vi "Tausand AB1000 Acquisition Example.vi"() -> ()   [LabVIEW 2015]
doc: "Example of a complete acquisition system using a Tausand Abacus.\n\nIncludes device identification, live settings changes and live data reading.\nData is shown in tables, graphs and saved in plain text files.\nUses a producer-consumer design pattern."
uses:
  <instrlib>/Tausand AB1000/Examples/sub vi/connectionState.ctl
  <instrlib>/Tausand AB1000/Public/Controls/settings4ch.ctl
  <instrlib>/Tausand AB1000/Public/Controls/configMultipleCoincRing.ctl
  <instrlib>/Tausand AB1000/Examples/sub vi/defaultSettings.ctl
  <instrlib>/Tausand AB1000/Public/Controls/deviceTypeRing.ctl
  <instrlib>/Tausand AB1000/Public/Controls/settings2ch.ctl
  <instrlib>/Tausand AB1000/Public/Controls/counters2ch.ctl
  <instrlib>/Tausand AB1000/Public/Controls/counters4ch.ctl
  <vilib>/Utility/miscctls.llb/LVRowAndColumnUnsignedTypeDef.ctl
  <instrlib>/Tausand AB1000/Public/Controls/channelRing.ctl
  <vilib>/Utility/file.llb/Write Delimited Spreadsheet (string).vi
  <vilib>/Utility/file.llb/Read Delimited Spreadsheet (string).vi
  <instrlib>/Tausand AB1000/Tausand AB1000.lvlib
panel:
  out "ref ctrls":T1
  out "timer-settings 2":timestamp
  in  "butLoadDefSett":bool
  out "ref indics":T2
  out "dafafile header":string[](array[string])
  in  "settings 2ch":T3={"sampling"=1000, "coincidence_window"=10, "delay_A"=0, "delay_B"=0, "sleep_A"=0, "sleep_B"=0} {"sleep_B" max=100 step=5; "sleep_A" max=100 step=5; "delay_B" max=100 step=5; "delay_A" max=100 step=5; "coincidence_window" min=1 max=50000 step=5; "sampling" items=["1ms"=1, "2ms"=2, "5ms"=5, "10ms"=10, "20ms"=20, "50ms"=50, "100ms"=100, "200ms"=200, "500ms"=500, "1s"=1000, "2s"=2000, "5s"=5000, "10s"=10000, "20s"=20000, "50s"=50000, "100s"=100000, "200s"=200000, "500s"=500000, "1000s"=1000000]}
  in  "settings 4ch":T4={"sampling"=1000, "coincidence_window"=10, "delay_A"=0, "delay_B"=0, "delay_C"=0, "delay_D"=0, "sleep_A"=0, "sleep_B"=0, "sleep_C"=0, "sleep_D"=0, "config_multiple_1"=240} {"config_multiple_1" items=["ABC"=224, "ABD"=208, "ACD"=176, "BCD"=112, "ABCD"=240]; "sleep_D" max=100 step=5; "sleep_C" max=100 step=5; "sleep_B" max=100 step=5; "sleep_A" max=100 step=5; "delay_D" max=100 step=5; "delay_C" max=100 step=5; "delay_B" max=100 step=5; "delay_A" max=100 step=5; "coincidence_window" min=1 max=10000 step=5; "sampling" items=["1ms"=1, "2ms"=2, "3ms"=3, "4ms"=4, "5ms"=5, "6ms"=6, "7ms"=7, "8ms"=8, "9ms"=9, "10ms"=10, "11ms"=11, "12ms"=12, "13ms"=13, "14ms"=14, "15ms"=15, "16ms"=16, "17ms"=17, "18ms"=18, "19ms"=19, "20ms"=20, "21ms"=21, "22ms"=22, "23ms"=23, "24ms"=24, "25ms"=25, "26ms"=26, "27ms"=27, "28ms"=28, "29ms"=29, "30ms"=30, "31ms"=31, "32ms"=32, "33ms"=33, "34ms"=34, "35ms"=35, "36ms"=36, "37ms"=37, "38ms"=38, "39ms"=39, "40ms"=40, "41ms"=41, "42ms"=42, "43ms"=43, "44ms"=44, "45ms"=45, "46ms"=46, "47ms"=47, "48ms"=48, "49ms"=49, "50ms"=50, "51ms"=51, "52ms"=52, "53ms"=53, "54ms"=54, "55ms"=55, "56ms"=56, "57ms"=57, "58ms"=58, "59ms"=59, "60ms"=60, "61ms"=61, "62ms"=62, "63ms"=63, "64ms"=64, "65ms"=65, "66ms"=66, "67ms"=67, "68ms"=68, "69ms"=69, "70ms"=70, "71ms"=71, "72ms"=72, "73ms"=73, "74ms"=74, "75ms"=75, "76ms"=76, "77ms"=77, "78ms"=78, "79ms"=79, "80ms"=80, "81ms"=81, "82ms"=82, "83ms"=83, "84ms"=84, "85ms"=85, "86ms"=86, "87ms"=87, "88ms"=88, "89ms"=89, "90ms"=90, "91ms"=91, "92ms"=92, "93ms"=93, "94ms"=94, "95ms"=95, "96ms"=96, "97ms"=97, "98ms"=98, "99ms"=99, "100ms"=100, "110ms"=110, "120ms"=120, "130ms"=130, "140ms"=140, "150ms"=150, "160ms"=160, "170ms"=170, "180ms"=180, "190ms"=190, "200ms"=200, "210ms"=210, "220ms"=220, "230ms"=230, "240ms"=240, "250ms"=250, "260ms"=260, "270ms"=270, "280ms"=280, "290ms"=290, "300ms"=300, "310ms"=310, "320ms"=320, "330ms"=330, "340ms"=340, "350ms"=350, "360ms"=360, "370ms"=370, "380ms"=380, "390ms"=390, "400ms"=400, "410ms"=410, "420ms"=420, "430ms"=430, "440ms"=440, "450ms"=450, "460ms"=460, "470ms"=470, "480ms"=480, "490ms"=490, "500ms"=500, "510ms"=510, "520ms"=520, "530ms"=530, "540ms"=540, "550ms"=550, "560ms"=560, "570ms"=570, "580ms"=580, "590ms"=590, "600ms"=600, "610ms"=610, "620ms"=620, "630ms"=630, "640ms"=640, "650ms"=650, "660ms"=660, "670ms"=670, "680ms"=680, "690ms"=690, "700ms"=700, "710ms"=710, "720ms"=720, "730ms"=730, "740ms"=740, "750ms"=750, "760ms"=760, "770ms"=770, "780ms"=780, "790ms"=790, "800ms"=800, "810ms"=810, "820ms"=820, "830ms"=830, "840ms"=840, "850ms"=850, "860ms"=860, "870ms"=870, "880ms"=880, "890ms"=890, "900ms"=900, "910ms"=910, "920ms"=920, "930ms"=930, "940ms"=940, "950ms"=950, "960ms"=960, "970ms"=970, "980ms"=980, "990ms"=990, "1,0s"=1000, "1,1s"=1100, "1,2s"=1200, "1,3s"=1300, "1,4s"=1400, "1,5s"=1500, "1,6s"=1600, "1,7s"=1700, "1,8s"=1800, "1,9s"=1900, "2,0s"=2000, "2,1s"=2100, "2,2s"=2200, "2,3s"=2300, "2,4s"=2400, "2,5s"=2500, "2,6s"=2600, "2,7s"=2700, "2,8s"=2800, "2,9s"=2900, "3,0s"=3000, "3,1s"=3100, "3,2s"=3200, "3,3s"=3300, "3,4s"=3400, "3,5s"=3500, "3,6s"=3600, "3,7s"=3700, "3,8s"=3800, "3,9s"=3900, "4,0s"=4000, "4,1s"=4100, "4,2s"=4200, "4,3s"=4300, "4,4s"=4400, "4,5s"=4500, "4,6s"=4600, "4,7s"=4700, "4,8s"=4800, "4,9s"=4900, "5,0s"=5000, "5,1s"=5100, "5,2s"=5200, "5,3s"=5300, "5,4s"=5400, "5,5s"=5500, "5,6s"=5600, "5,7s"=5700, "5,8s"=5800, "5,9s"=5900, "6,0s"=6000, "6,1s"=6100, "6,2s"=6200, "6,3s"=6300, "6,4s"=6400, "6,5s"=6500, "6,6s"=6600, "6,7s"=6700, "6,8s"=6800, "6,9s"=6900, "7,0s"=7000, "7,1s"=7100, "7,2s"=7200, "7,3s"=7300, "7,4s"=7400, "7,5s"=7500, "7,6s"=7600, "7,7s"=7700, "7,8s"=7800, "7,9s"=7900, "8,0s"=8000, "8,1s"=8100, "8,2s"=8200, "8,3s"=8300, "8,4s"=8400, "8,5s"=8500, "8,6s"=8600, "8,7s"=8700, "8,8s"=8800, "8,9s"=8900, "9,0s"=9000, "9,1s"=9100, "9,2s"=9200, "9,3s"=9300, "9,4s"=9400, "9,5s"=9500, "9,6s"=9600, "9,7s"=9700, "9,8s"=9800, "9,9s"=9900, "10s"=10000, "11s"=11000, "12s"=12000, "13s"=13000, "14s"=14000, "15s"=15000, "16s"=16000, "17s"=17000, "18s"=18000, "19s"=19000, "20s"=20000, "21s"=21000, "22s"=22000, "23s"=23000, "24s"=24000, "25s"=25000, "26s"=26000, "27s"=27000, "28s"=28000, "29s"=29000, "30s"=30000, "31s"=31000, "32s"=32000, "33s"=33000, "34s"=34000, "35s"=35000, "36s"=36000, "37s"=37000, "38s"=38000, "39s"=39000, "40s"=40000, "41s"=41000, "42s"=42000, "43s"=43000, "44s"=44000, "45s"=45000, "46s"=46000, "47s"=47000, "48s"=48000, "49s"=49000, "50s"=50000, "51s"=51000, "52s"=52000, "53s"=53000, "54s"=54000, "55s"=55000, "56s"=56000, "57s"=57000, "58s"=58000, "59s"=59000, "60s"=60000, "61s"=61000, "62s"=62000, "63s"=63000, "64s"=64000, "65s"=65000, "66s"=66000, "67s"=67000, "68s"=68000, "69s"=69000, "70s"=70000, "71s"=71000, "72s"=72000, "73s"=73000, "74s"=74000, "75s"=75000, "76s"=76000, "77s"=77000, "78s"=78000, "79s"=79000, "80s"=80000, "81s"=81000, "82s"=82000, "83s"=83000, "84s"=84000, "85s"=85000, "86s"=86000, "87s"=87000, "88s"=88000, "89s"=89000, "90s"=90000, "91s"=91000, "92s"=92000, "93s"=93000, "94s"=94000, "95s"=95000, "96s"=96000, "97s"=97000, "98s"=98000, "99s"=99000, "100s"=100000, "110s"=110000, "120s"=120000, "130s"=130000, "140s"=140000, "150s"=150000, "160s"=160000, "170s"=170000, "180s"=180000, "190s"=190000, "200s"=200000, "210s"=210000, "220s"=220000, "230s"=230000, "240s"=240000, "250s"=250000, "260s"=260000, "270s"=270000, "280s"=280000, "290s"=290000, "300s"=300000, "310s"=310000, "320s"=320000, "330s"=330000, "340s"=340000, "350s"=350000, "360s"=360000, "370s"=370000, "380s"=380000, "390s"=390000, "400s"=400000, "410s"=410000, "420s"=420000, "430s"=430000, "440s"=440000, "450s"=450000, "460s"=460000, "470s"=470000, "480s"=480000, "490s"=490000, "500s"=500000, "510s"=510000, "520s"=520000, "530s"=530000, "540s"=540000, "550s"=550000, "560s"=560000, "570s"=570000, "580s"=580000, "590s"=590000, "600s"=600000, "610s"=610000, "620s"=620000, "630s"=630000, "640s"=640000, "650s"=650000, "660s"=660000, "670s"=670000, "680s"=680000, "690s"=690000, "700s"=700000, "710s"=710000, "720s"=720000, "730s"=730000, "740s"=740000, "750s"=750000, "760s"=760000, "770s"=770000, "780s"=780000, "790s"=790000, "800s"=800000, "810s"=810000, "820s"=820000, "830s"=830000, "840s"=840000, "850s"=850000, "860s"=860000, "870s"=870000, "880s"=880000, "890s"=890000, "900s"=900000, "910s"=910000, "920s"=920000, "930s"=930000, "940s"=940000, "950s"=950000, "960s"=960000, "970s"=970000, "980s"=980000, "990s"=990000, "1000s"=1000000]}
  out "device type":T6 items=["any"=0, "AB1002"=1002, "AB1004"=1004, "AB1502"=1502, "AB1504"=1504, "AB2002"=2002, "AB2004"=2004, "AB2502"=2502, "AB2504"=2504]
  out "path-defsettings":path
  out "delimiter":string
  out "default settings":T7={"autogenerate"=FALSE, "datetime"=FALSE, "from_device"=FALSE, "directory"="", "file_prefix"="", "settings_suffix"="", "delimiter"="", "extension"="", "Abacus settings"={"sampling"=0, "coincidence_window"=0, "delay_A"=0, "delay_B"=0, "delay_C"=0, "delay_D"=0, "sleep_A"=0, "sleep_B"=0, "sleep_C"=0, "sleep_D"=0, "config_multiple_1"=240}} {"Abacus settings"."config_multiple_1" items=["ABC"=224, "ABD"=208, "ACD"=176, "BCD"=112, "ABCD"=240]; "Abacus settings"."sleep_D" max=100 step=5; "Abacus settings"."sleep_C" max=100 step=5; "Abacus settings"."sleep_B" max=100 step=5; "Abacus settings"."sleep_A" max=100 step=5; "Abacus settings"."delay_D" max=100 step=5; "Abacus settings"."delay_C" max=100 step=5; "Abacus settings"."delay_B" max=100 step=5; "Abacus settings"."delay_A" max=100 step=5; "Abacus settings"."coincidence_window" min=5 max=10000 step=5; "Abacus settings"."sampling" items=["1ms"=1, "2ms"=2, "3ms"=3, "4ms"=4, "5ms"=5, "6ms"=6, "7ms"=7, "8ms"=8, "9ms"=9, "10ms"=10, "11ms"=11, "12ms"=12, "13ms"=13, "14ms"=14, "15ms"=15, "16ms"=16, "17ms"=17, "18ms"=18, "19ms"=19, "20ms"=20, "21ms"=21, "22ms"=22, "23ms"=23, "24ms"=24, "25ms"=25, "26ms"=26, "27ms"=27, "28ms"=28, "29ms"=29, "30ms"=30, "31ms"=31, "32ms"=32, "33ms"=33, "34ms"=34, "35ms"=35, "36ms"=36, "37ms"=37, "38ms"=38, "39ms"=39, "40ms"=40, "41ms"=41, "42ms"=42, "43ms"=43, "44ms"=44, "45ms"=45, "46ms"=46, "47ms"=47, "48ms"=48, "49ms"=49, "50ms"=50, "51ms"=51, "52ms"=52, "53ms"=53, "54ms"=54, "55ms"=55, "56ms"=56, "57ms"=57, "58ms"=58, "59ms"=59, "60ms"=60, "61ms"=61, "62ms"=62, "63ms"=63, "64ms"=64, "65ms"=65, "66ms"=66, "67ms"=67, "68ms"=68, "69ms"=69, "70ms"=70, "71ms"=71, "72ms"=72, "73ms"=73, "74ms"=74, "75ms"=75, "76ms"=76, "77ms"=77, "78ms"=78, "79ms"=79, "80ms"=80, "81ms"=81, "82ms"=82, "83ms"=83, "84ms"=84, "85ms"=85, "86ms"=86, "87ms"=87, "88ms"=88, "89ms"=89, "90ms"=90, "91ms"=91, "92ms"=92, "93ms"=93, "94ms"=94, "95ms"=95, "96ms"=96, "97ms"=97, "98ms"=98, "99ms"=99, "100ms"=100, "110ms"=110, "120ms"=120, "130ms"=130, "140ms"=140, "150ms"=150, "160ms"=160, "170ms"=170, "180ms"=180, "190ms"=190, "200ms"=200, "210ms"=210, "220ms"=220, "230ms"=230, "240ms"=240, "250ms"=250, "260ms"=260, "270ms"=270, "280ms"=280, "290ms"=290, "300ms"=300, "310ms"=310, "320ms"=320, "330ms"=330, "340ms"=340, "350ms"=350, "360ms"=360, "370ms"=370, "380ms"=380, "390ms"=390, "400ms"=400, "410ms"=410, "420ms"=420, "430ms"=430, "440ms"=440, "450ms"=450, "460ms"=460, "470ms"=470, "480ms"=480, "490ms"=490, "500ms"=500, "510ms"=510, "520ms"=520, "530ms"=530, "540ms"=540, "550ms"=550, "560ms"=560, "570ms"=570, "580ms"=580, "590ms"=590, "600ms"=600, "610ms"=610, "620ms"=620, "630ms"=630, "640ms"=640, "650ms"=650, "660ms"=660, "670ms"=670, "680ms"=680, "690ms"=690, "700ms"=700, "710ms"=710, "720ms"=720, "730ms"=730, "740ms"=740, "750ms"=750, "760ms"=760, "770ms"=770, "780ms"=780, "790ms"=790, "800ms"=800, "810ms"=810, "820ms"=820, "830ms"=830, "840ms"=840, "850ms"=850, "860ms"=860, "870ms"=870, "880ms"=880, "890ms"=890, "900ms"=900, "910ms"=910, "920ms"=920, "930ms"=930, "940ms"=940, "950ms"=950, "960ms"=960, "970ms"=970, "980ms"=980, "990ms"=990, "1,0s"=1000, "1,1s"=1100, "1,2s"=1200, "1,3s"=1300, "1,4s"=1400, "1,5s"=1500, "1,6s"=1600, "1,7s"=1700, "1,8s"=1800, "1,9s"=1900, "2,0s"=2000, "2,1s"=2100, "2,2s"=2200, "2,3s"=2300, "2,4s"=2400, "2,5s"=2500, "2,6s"=2600, "2,7s"=2700, "2,8s"=2800, "2,9s"=2900, "3,0s"=3000, "3,1s"=3100, "3,2s"=3200, "3,3s"=3300, "3,4s"=3400, "3,5s"=3500, "3,6s"=3600, "3,7s"=3700, "3,8s"=3800, "3,9s"=3900, "4,0s"=4000, "4,1s"=4100, "4,2s"=4200, "4,3s"=4300, "4,4s"=4400, "4,5s"=4500, "4,6s"=4600, "4,7s"=4700, "4,8s"=4800, "4,9s"=4900, "5,0s"=5000, "5,1s"=5100, "5,2s"=5200, "5,3s"=5300, "5,4s"=5400, "5,5s"=5500, "5,6s"=5600, "5,7s"=5700, "5,8s"=5800, "5,9s"=5900, "6,0s"=6000, "6,1s"=6100, "6,2s"=6200, "6,3s"=6300, "6,4s"=6400, "6,5s"=6500, "6,6s"=6600, "6,7s"=6700, "6,8s"=6800, "6,9s"=6900, "7,0s"=7000, "7,1s"=7100, "7,2s"=7200, "7,3s"=7300, "7,4s"=7400, "7,5s"=7500, "7,6s"=7600, "7,7s"=7700, "7,8s"=7800, "7,9s"=7900, "8,0s"=8000, "8,1s"=8100, "8,2s"=8200, "8,3s"=8300, "8,4s"=8400, "8,5s"=8500, "8,6s"=8600, "8,7s"=8700, "8,8s"=8800, "8,9s"=8900, "9,0s"=9000, "9,1s"=9100, "9,2s"=9200, "9,3s"=9300, "9,4s"=9400, "9,5s"=9500, "9,6s"=9600, "9,7s"=9700, "9,8s"=9800, "9,9s"=9900, "10s"=10000, "11s"=11000, "12s"=12000, "13s"=13000, "14s"=14000, "15s"=15000, "16s"=16000, "17s"=17000, "18s"=18000, "19s"=19000, "20s"=20000, "21s"=21000, "22s"=22000, "23s"=23000, "24s"=24000, "25s"=25000, "26s"=26000, "27s"=27000, "28s"=28000, "29s"=29000, "30s"=30000, "31s"=31000, "32s"=32000, "33s"=33000, "34s"=34000, "35s"=35000, "36s"=36000, "37s"=37000, "38s"=38000, "39s"=39000, "40s"=40000, "41s"=41000, "42s"=42000, "43s"=43000, "44s"=44000, "45s"=45000, "46s"=46000, "47s"=47000, "48s"=48000, "49s"=49000, "50s"=50000, "51s"=51000, "52s"=52000, "53s"=53000, "54s"=54000, "55s"=55000, "56s"=56000, "57s"=57000, "58s"=58000, "59s"=59000, "60s"=60000, "61s"=61000, "62s"=62000, "63s"=63000, "64s"=64000, "65s"=65000, "66s"=66000, "67s"=67000, "68s"=68000, "69s"=69000, "70s"=70000, "71s"=71000, "72s"=72000, "73s"=73000, "74s"=74000, "75s"=75000, "76s"=76000, "77s"=77000, "78s"=78000, "79s"=79000, "80s"=80000, "81s"=81000, "82s"=82000, "83s"=83000, "84s"=84000, "85s"=85000, "86s"=86000, "87s"=87000, "88s"=88000, "89s"=89000, "90s"=90000, "91s"=91000, "92s"=92000, "93s"=93000, "94s"=94000, "95s"=95000, "96s"=96000, "97s"=97000, "98s"=98000, "99s"=99000, "100s"=100000, "110s"=110000, "120s"=120000, "130s"=130000, "140s"=140000, "150s"=150000, "160s"=160000, "170s"=170000, "180s"=180000, "190s"=190000, "200s"=200000, "210s"=210000, "220s"=220000, "230s"=230000, "240s"=240000, "250s"=250000, "260s"=260000, "270s"=270000, "280s"=280000, "290s"=290000, "300s"=300000, "310s"=310000, "320s"=320000, "330s"=330000, "340s"=340000, "350s"=350000, "360s"=360000, "370s"=370000, "380s"=380000, "390s"=390000, "400s"=400000, "410s"=410000, "420s"=420000, "430s"=430000, "440s"=440000, "450s"=450000, "460s"=460000, "470s"=470000, "480s"=480000, "490s"=490000, "500s"=500000, "510s"=510000, "520s"=520000, "530s"=530000, "540s"=540000, "550s"=550000, "560s"=560000, "570s"=570000, "580s"=580000, "590s"=590000, "600s"=600000, "610s"=610000, "620s"=620000, "630s"=630000, "640s"=640000, "650s"=650000, "660s"=660000, "670s"=670000, "680s"=680000, "690s"=690000, "700s"=700000, "710s"=710000, "720s"=720000, "730s"=730000, "740s"=740000, "750s"=750000, "760s"=760000, "770s"=770000, "780s"=780000, "790s"=790000, "800s"=800000, "810s"=810000, "820s"=820000, "830s"=830000, "840s"=840000, "850s"=850000, "860s"=860000, "870s"=870000, "880s"=880000, "890s"=890000, "900s"=900000, "910s"=910000, "920s"=920000, "930s"=930000, "940s"=940000, "950s"=950000, "960s"=960000, "970s"=970000, "980s"=980000, "990s"=990000, "1000s"=1000000]}
  out "settings_old":T4={"sampling"=1000, "coincidence_window"=10, "delay_A"=0, "delay_B"=0, "delay_C"=0, "delay_D"=0, "sleep_A"=0, "sleep_B"=0, "sleep_C"=0, "sleep_D"=0, "config_multiple_1"=0} {"config_multiple_1" items=["ABC"=224, "ABD"=208, "ACD"=176, "BCD"=112, "ABCD"=240]; "sleep_D" max=100 step=1; "sleep_C" max=100 step=1; "sleep_B" max=100 step=1; "sleep_A" max=100 step=1; "delay_D" max=100 step=1; "delay_C" max=100 step=1; "delay_B" max=100 step=1; "delay_A" max=100 step=1; "coincidence_window" min=1 max=10000 step=1; "sampling" items=["1ms"=1, "2ms"=2, "3ms"=3, "4ms"=4, "5ms"=5, "6ms"=6, "7ms"=7, "8ms"=8, "9ms"=9, "10ms"=10, "11ms"=11, "12ms"=12, "13ms"=13, "14ms"=14, "15ms"=15, "16ms"=16, "17ms"=17, "18ms"=18, "19ms"=19, "20ms"=20, "21ms"=21, "22ms"=22, "23ms"=23, "24ms"=24, "25ms"=25, "26ms"=26, "27ms"=27, "28ms"=28, "29ms"=29, "30ms"=30, "31ms"=31, "32ms"=32, "33ms"=33, "34ms"=34, "35ms"=35, "36ms"=36, "37ms"=37, "38ms"=38, "39ms"=39, "40ms"=40, "41ms"=41, "42ms"=42, "43ms"=43, "44ms"=44, "45ms"=45, "46ms"=46, "47ms"=47, "48ms"=48, "49ms"=49, "50ms"=50, "51ms"=51, "52ms"=52, "53ms"=53, "54ms"=54, "55ms"=55, "56ms"=56, "57ms"=57, "58ms"=58, "59ms"=59, "60ms"=60, "61ms"=61, "62ms"=62, "63ms"=63, "64ms"=64, "65ms"=65, "66ms"=66, "67ms"=67, "68ms"=68, "69ms"=69, "70ms"=70, "71ms"=71, "72ms"=72, "73ms"=73, "74ms"=74, "75ms"=75, "76ms"=76, "77ms"=77, "78ms"=78, "79ms"=79, "80ms"=80, "81ms"=81, "82ms"=82, "83ms"=83, "84ms"=84, "85ms"=85, "86ms"=86, "87ms"=87, "88ms"=88, "89ms"=89, "90ms"=90, "91ms"=91, "92ms"=92, "93ms"=93, "94ms"=94, "95ms"=95, "96ms"=96, "97ms"=97, "98ms"=98, "99ms"=99, "100ms"=100, "110ms"=110, "120ms"=120, "130ms"=130, "140ms"=140, "150ms"=150, "160ms"=160, "170ms"=170, "180ms"=180, "190ms"=190, "200ms"=200, "210ms"=210, "220ms"=220, "230ms"=230, "240ms"=240, "250ms"=250, "260ms"=260, "270ms"=270, "280ms"=280, "290ms"=290, "300ms"=300, "310ms"=310, "320ms"=320, "330ms"=330, "340ms"=340, "350ms"=350, "360ms"=360, "370ms"=370, "380ms"=380, "390ms"=390, "400ms"=400, "410ms"=410, "420ms"=420, "430ms"=430, "440ms"=440, "450ms"=450, "460ms"=460, "470ms"=470, "480ms"=480, "490ms"=490, "500ms"=500, "510ms"=510, "520ms"=520, "530ms"=530, "540ms"=540, "550ms"=550, "560ms"=560, "570ms"=570, "580ms"=580, "590ms"=590, "600ms"=600, "610ms"=610, "620ms"=620, "630ms"=630, "640ms"=640, "650ms"=650, "660ms"=660, "670ms"=670, "680ms"=680, "690ms"=690, "700ms"=700, "710ms"=710, "720ms"=720, "730ms"=730, "740ms"=740, "750ms"=750, "760ms"=760, "770ms"=770, "780ms"=780, "790ms"=790, "800ms"=800, "810ms"=810, "820ms"=820, "830ms"=830, "840ms"=840, "850ms"=850, "860ms"=860, "870ms"=870, "880ms"=880, "890ms"=890, "900ms"=900, "910ms"=910, "920ms"=920, "930ms"=930, "940ms"=940, "950ms"=950, "960ms"=960, "970ms"=970, "980ms"=980, "990ms"=990, "1,0s"=1000, "1,1s"=1100, "1,2s"=1200, "1,3s"=1300, "1,4s"=1400, "1,5s"=1500, "1,6s"=1600, "1,7s"=1700, "1,8s"=1800, "1,9s"=1900, "2,0s"=2000, "2,1s"=2100, "2,2s"=2200, "2,3s"=2300, "2,4s"=2400, "2,5s"=2500, "2,6s"=2600, "2,7s"=2700, "2,8s"=2800, "2,9s"=2900, "3,0s"=3000, "3,1s"=3100, "3,2s"=3200, "3,3s"=3300, "3,4s"=3400, "3,5s"=3500, "3,6s"=3600, "3,7s"=3700, "3,8s"=3800, "3,9s"=3900, "4,0s"=4000, "4,1s"=4100, "4,2s"=4200, "4,3s"=4300, "4,4s"=4400, "4,5s"=4500, "4,6s"=4600, "4,7s"=4700, "4,8s"=4800, "4,9s"=4900, "5,0s"=5000, "5,1s"=5100, "5,2s"=5200, "5,3s"=5300, "5,4s"=5400, "5,5s"=5500, "5,6s"=5600, "5,7s"=5700, "5,8s"=5800, "5,9s"=5900, "6,0s"=6000, "6,1s"=6100, "6,2s"=6200, "6,3s"=6300, "6,4s"=6400, "6,5s"=6500, "6,6s"=6600, "6,7s"=6700, "6,8s"=6800, "6,9s"=6900, "7,0s"=7000, "7,1s"=7100, "7,2s"=7200, "7,3s"=7300, "7,4s"=7400, "7,5s"=7500, "7,6s"=7600, "7,7s"=7700, "7,8s"=7800, "7,9s"=7900, "8,0s"=8000, "8,1s"=8100, "8,2s"=8200, "8,3s"=8300, "8,4s"=8400, "8,5s"=8500, "8,6s"=8600, "8,7s"=8700, "8,8s"=8800, "8,9s"=8900, "9,0s"=9000, "9,1s"=9100, "9,2s"=9200, "9,3s"=9300, "9,4s"=9400, "9,5s"=9500, "9,6s"=9600, "9,7s"=9700, "9,8s"=9800, "9,9s"=9900, "10s"=10000, "11s"=11000, "12s"=12000, "13s"=13000, "14s"=14000, "15s"=15000, "16s"=16000, "17s"=17000, "18s"=18000, "19s"=19000, "20s"=20000, "21s"=21000, "22s"=22000, "23s"=23000, "24s"=24000, "25s"=25000, "26s"=26000, "27s"=27000, "28s"=28000, "29s"=29000, "30s"=30000, "31s"=31000, "32s"=32000, "33s"=33000, "34s"=34000, "35s"=35000, "36s"=36000, "37s"=37000, "38s"=38000, "39s"=39000, "40s"=40000, "41s"=41000, "42s"=42000, "43s"=43000, "44s"=44000, "45s"=45000, "46s"=46000, "47s"=47000, "48s"=48000, "49s"=49000, "50s"=50000, "51s"=51000, "52s"=52000, "53s"=53000, "54s"=54000, "55s"=55000, "56s"=56000, "57s"=57000, "58s"=58000, "59s"=59000, "60s"=60000, "61s"=61000, "62s"=62000, "63s"=63000, "64s"=64000, "65s"=65000, "66s"=66000, "67s"=67000, "68s"=68000, "69s"=69000, "70s"=70000, "71s"=71000, "72s"=72000, "73s"=73000, "74s"=74000, "75s"=75000, "76s"=76000, "77s"=77000, "78s"=78000, "79s"=79000, "80s"=80000, "81s"=81000, "82s"=82000, "83s"=83000, "84s"=84000, "85s"=85000, "86s"=86000, "87s"=87000, "88s"=88000, "89s"=89000, "90s"=90000, "91s"=91000, "92s"=92000, "93s"=93000, "94s"=94000, "95s"=95000, "96s"=96000, "97s"=97000, "98s"=98000, "99s"=99000, "100s"=100000, "110s"=110000, "120s"=120000, "130s"=130000, "140s"=140000, "150s"=150000, "160s"=160000, "170s"=170000, "180s"=180000, "190s"=190000, "200s"=200000, "210s"=210000, "220s"=220000, "230s"=230000, "240s"=240000, "250s"=250000, "260s"=260000, "270s"=270000, "280s"=280000, "290s"=290000, "300s"=300000, "310s"=310000, "320s"=320000, "330s"=330000, "340s"=340000, "350s"=350000, "360s"=360000, "370s"=370000, "380s"=380000, "390s"=390000, "400s"=400000, "410s"=410000, "420s"=420000, "430s"=430000, "440s"=440000, "450s"=450000, "460s"=460000, "470s"=470000, "480s"=480000, "490s"=490000, "500s"=500000, "510s"=510000, "520s"=520000, "530s"=530000, "540s"=540000, "550s"=550000, "560s"=560000, "570s"=570000, "580s"=580000, "590s"=590000, "600s"=600000, "610s"=610000, "620s"=620000, "630s"=630000, "640s"=640000, "650s"=650000, "660s"=660000, "670s"=670000, "680s"=680000, "690s"=690000, "700s"=700000, "710s"=710000, "720s"=720000, "730s"=730000, "740s"=740000, "750s"=750000, "760s"=760000, "770s"=770000, "780s"=780000, "790s"=790000, "800s"=800000, "810s"=810000, "820s"=820000, "830s"=830000, "840s"=840000, "850s"=850000, "860s"=860000, "870s"=870000, "880s"=880000, "890s"=890000, "900s"=900000, "910s"=910000, "920s"=920000, "930s"=930000, "940s"=940000, "950s"=950000, "960s"=960000, "970s"=970000, "980s"=980000, "990s"=990000, "1000s"=1000000]}
  out "sttgs changed?":bool[](array[boolean])
  out "connection state":T8
  out "timer-reconnect":timestamp
  out "status":string
  out "path-new":path
  out "error":errorcluster
  out "path-settingsOld":path
  out "path-settings":path
  out "timer-settings":timestamp
  out "timer-readRequest":timestamp
  in  "Tab Control":T9(tab)
  out "dataTable":string[][](table)
  out "counters 2ch":T10
  out "counters 4ch":T11
  out "graph-A":cluster{timestamp[], u32[]}(graph) caption="small graph A"
  out "graph-B":cluster{timestamp[], u32[]}(graph) caption="small graph B"
  out "graph-C":cluster{timestamp[], u32[]}(graph) caption="small graph C"
  out "graph-D":cluster{timestamp[], u32[]}(graph) caption="small graph D"
  out "graph coinc":cluster{timestamp[], u32[]}[](graph)
  out "graph-A-S":cluster{timestamp[], u32[]}(graph) caption="small graph A"
  out "graph-B-S":cluster{timestamp[], u32[]}(graph) caption="small graph B"
  out "graph-C-S":cluster{timestamp[], u32[]}(graph) caption="small graph C"
  out "graph-D-S":cluster{timestamp[], u32[]}(graph) caption="small graph D"
  in  "butDisconnect":bool
  in  "butConnect":bool
  in  "butUnlockSett":bool
  in  "butStopAcq":bool
  in  "butStartAcq":bool
  out "path-fileOld":path
  in  "path-file":path caption="Save as"
  out "timer-begin":timestamp
  out "timer-nextRead":timestamp
  out "timer-lastRead":timestamp
  out "timer-current":timestamp
  out "abacus VISA":refnum<visa-resource-name>
  in  "butExit":bool
  # "Settings"
  # "January 2023"
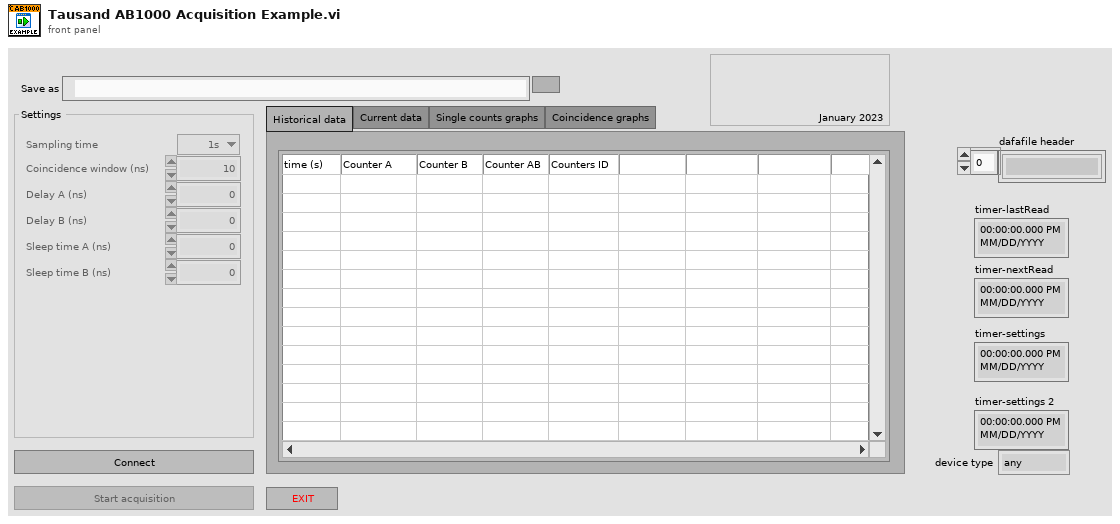
[diagram p1: front panel]
types:
  T1 = cluster{"butConnect":refnum<vi>, "butDisconnect":refnum<vi>, "butStartAcq":refnum<vi>, "butStopAcq":refnum<vi>, "butLoadDefSett":refnum<vi>, "butUnlockSett":refnum<vi>, "settings 2ch":refnum<vi>, "settings 4ch":refnum<vi>}
  T2 = cluster{"counters 2ch":refnum<vi>, "counters 4ch":refnum<vi>, "dataTable":refnum<vi>, "graph coinc":refnum<vi>, "graph-A":refnum<vi>, "graph-A-S":refnum<vi>, "graph-B":refnum<vi>, "graph-B-S":refnum<vi>, "graph-C":refnum<vi>, "graph-C-S":refnum<vi>, "graph-D":refnum<vi>, "graph-D-S":refnum<vi>}
  T3 = typedef "Tausand AB1000.lvlib/settings2ch.ctl" = cluster{"sampling":u32, "coincidence_window":u32, "delay_A":u32, "delay_B":u32, "sleep_A":u32, "sleep_B":u32}
  T4 = typedef "Tausand AB1000.lvlib/settings4ch.ctl" = cluster{"sampling":u32, "coincidence_window":u32, "delay_A":u32, "delay_B":u32, "delay_C":u32, "delay_D":u32, "sleep_A":u32, "sleep_B":u32, "sleep_C":u32, "sleep_D":u32, "config_multiple_1":T5}
  T5 = typedef "Tausand AB1000.lvlib/configMultipleCoincRing.ctl" = u16
  T6 = typedef "Tausand AB1000.lvlib/deviceTypeRing.ctl" = u16
  T7 = typedef "defaultSettings.ctl" = cluster{"autogenerate":bool, "datetime":bool, "from_device":bool, "directory":string, "file_prefix":string, "settings_suffix":string, "delimiter":string, "extension":string, "Abacus settings":T4}
  T8 = typedef "connectionState.ctl" = enum16{"disconnected", "connected", "acquiring data", "connection error", "acquisition error"}
  T9 = enum32{"Historical data", "Current data", "Single counts graphs", "Coincidence graphs"}
  T10 = typedef "Tausand AB1000.lvlib/counters2ch.ctl" = cluster{"counter_A":u32, "counter_B":u32, "counter_AB":u32, "counters_ID":u32, "time_left":u32}
  T11 = typedef "Tausand AB1000.lvlib/counters4ch.ctl" = cluster{"counter_A":u32, "counter_B":u32, "counter_C":u32, "counter_D":u32, "counter_AB":u32, "counter_AC":u32, "counter_AD":u32, "counter_BC":u32, "counter_BD":u32, "counter_CD":u32, "counter_multiple_1":u32, "counters_ID":u32, "time_left":u32}
  T12 = cluster{"seconds since 1Jan1904":timestamp, "counters 4ch":T11}[]
  T13 = typedef "Semaphore RefNum" = refnum<k1>
  T14 = cluster{"semaphore files":T13, "semaphore port":T13, "notifier read request":refnum<notifier>, "queue data":refnum<queue>, "queue instructions":refnum<queue>}
  T15 = cluster{"seconds since 1Jan1904":timestamp, "counters 4ch":T11}
  T16 = cluster{"sampling":bool, "coincidence_window":bool, "delay_A":bool, "delay_B":bool, "delay_C":bool, "delay_D":bool, "sleep_A":bool, "sleep_B":bool, "sleep_C":bool, "sleep_D":bool, "config_multiple_1":bool}
  T17 = enum8{"Enabled", "Disabled", "Disabled and Grayed Out"}
  T18 = cluster{"counter_A":u32, "counter_B":u32, "counter_C":u32, "counter_D":u32, "counter_AB":u32, "counter_AC":u32, "counter_AD":u32, "counter_BC":u32, "counter_BD":u32, "counter_CD":u32, "counter_multiple_1":u32, "counters_ID":u32, "time_left":u32}
  T19 = typedef "LVRowAndColumnUnsignedTypeDef.ctl" = cluster{"Row":u32, "Column":u32}
  T20 = cluster{"[0]":u32, "[1]":u32, "[2]":u32, "[3]":u32, "[4]":u32, "[5]":u32, "[6]":u32, "[7]":u32, "[8]":u32, "[9]":u32, "[10]":u32}
  T21 = typedef "abacus4ch.lvlib/settings4ch.ctl" = cluster{"sampling":u32, "coincidence_window":u32, "delay_A":u32, "delay_B":u32, "delay_C":u32, "delay_D":u32, "sleep_A":u32, "sleep_B":u32, "sleep_C":u32, "sleep_D":u32, "config_multiple_1":T22}
  T22 = typedef "abacus4ch.lvlib/configMultipleCoincRing.ctl" = u16
  T23 = typedef "Tausand AB1000.lvlib/channelRing.ctl" = u8
  T24 = cluster{"read time":timestamp, "output cluster 4ch":T11}
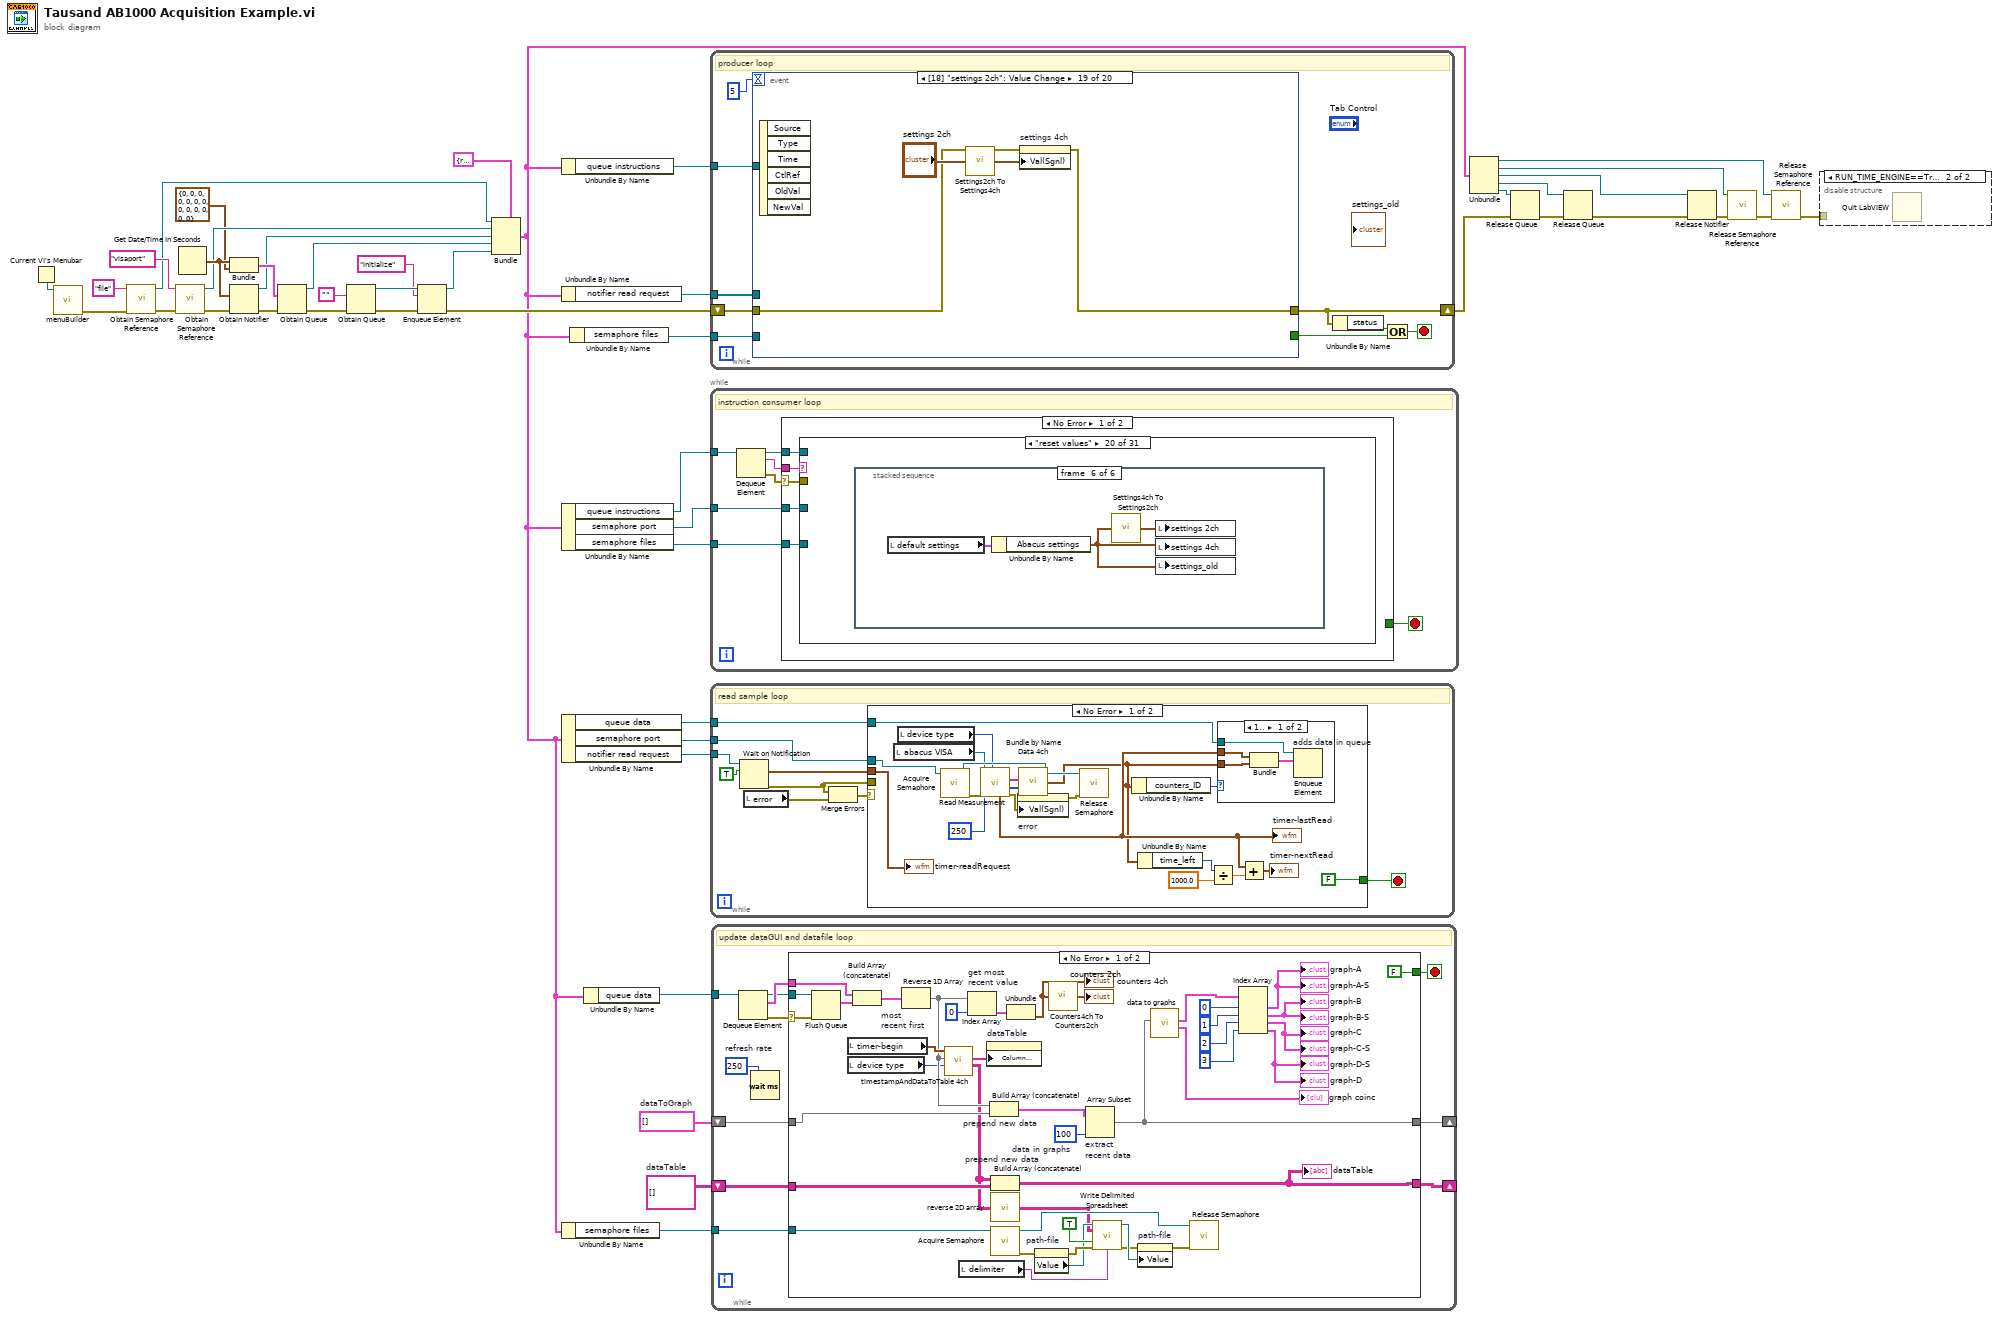
[diagram p0: block diagram]
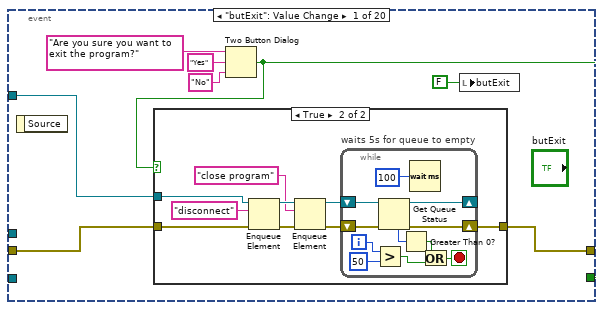
[diagram p2: hidden frame]
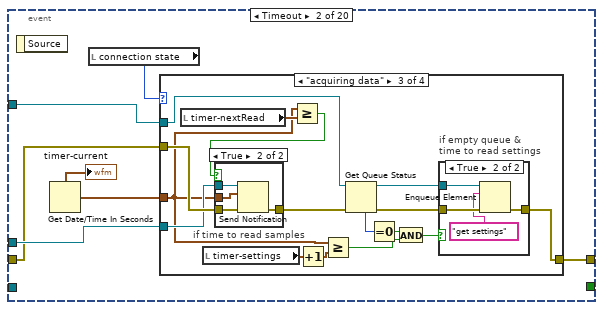
[diagram p4: hidden frame]
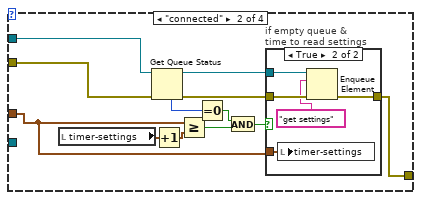
[diagram p6: hidden frame]
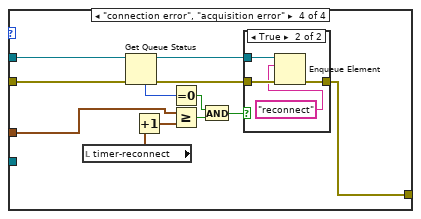
[diagram p10: hidden frame]
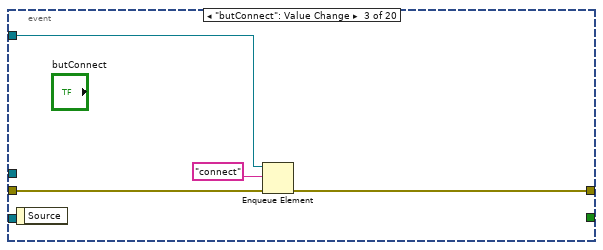
[diagram p12: hidden frame]
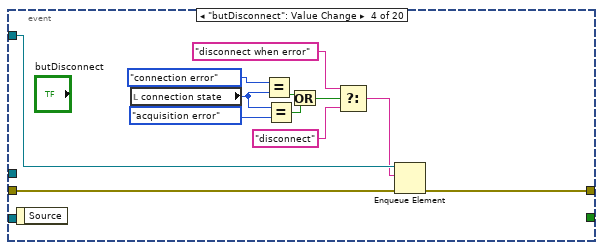
[diagram p13: hidden frame]
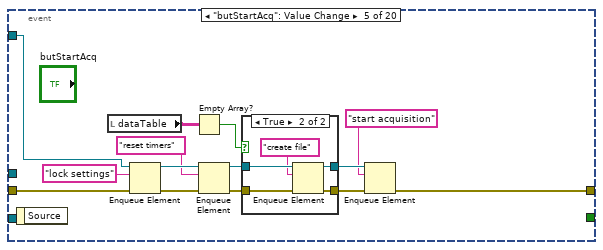
[diagram p14: hidden frame]
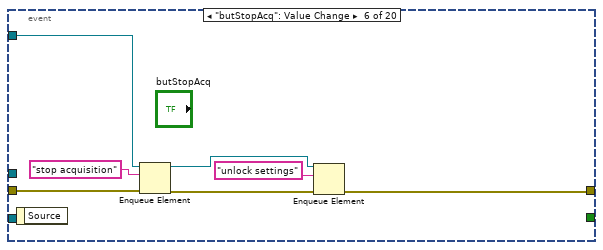
[diagram p16: hidden frame]
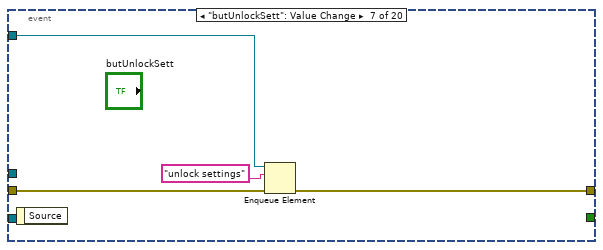
[diagram p17: hidden frame]
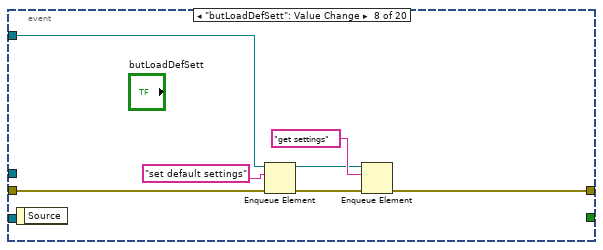
[diagram p18: hidden frame]
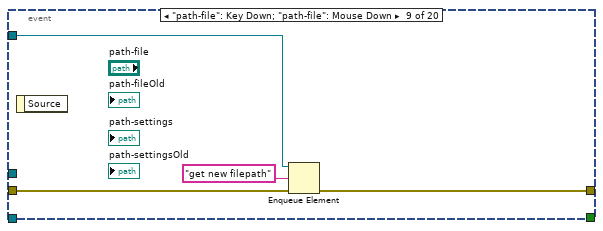
[diagram p19: hidden frame]
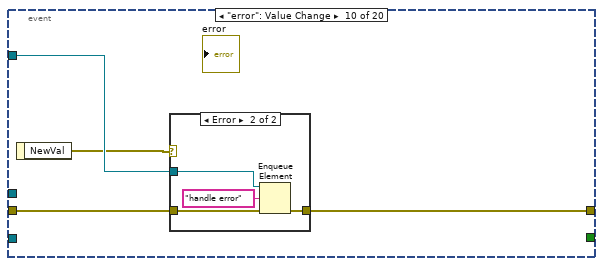
[diagram p20: hidden frame]
diagram:
  w1 = string[][] []  # dataTable
  w2 = T12 []  # dataToGraph
  n1 = Current VI's Menubar() -> (w7:refnum<k9>)
  n2 = call <instrlib>:"menuBuilder.vi"("Menu in"=w7) -> ("error out"=w8:errorcluster)  [unwired: 10 in]
  n3 = call <vilib>:"Obtain Semaphore Reference.vi"("error in (no error)"=w8, "name (unnamed)"="file") -> ("error out"=w34:errorcluster, "semaphore"=w13:T13)  [unwired: 3 in, 1 out]
  n4 = call <vilib>:"Obtain Semaphore Reference.vi"("error in (no error)"=w34, "name (unnamed)"="visaport") -> ("error out"=w37:errorcluster, "semaphore"=w32:T13)  [unwired: 3 in, 1 out]
  n5 = Get Date/Time In Seconds() -> (seconds since 1Jan1904=w36:timestamp)
  n6 = Bundle("seconds since 1Jan1904"=w36, "counters 4ch"=T11 {"counter_A"=0, "counter_B"=0, "counter_C"=0, "counter_D"=0, "counter_AB"=0, "counter_AC"=0, "counter_AD"=0, "counter_BC"=0, "counter_BD"=0, "counter_CD"=0, "counter_multiple_1"=0, "counters_ID"=0, "time_left"=0}) -> (w46:T15)  [unwired: 1 in]
  n7 = Obtain Notifier(notification data type=w36, error in (no error)=w37) -> (notifier out=w31:refnum<notifier>, error out=w45:errorcluster)  [unwired: 2 in, 1 out]
  n8 = Obtain Queue(element data type=w46, error in (no error)=w45) -> (queue out=w3:refnum<queue>, error out=w44:errorcluster)  [unwired: 3 in, 1 out]
  n9 = Obtain Queue(element data type="" ("str const"), error in (no error)=w44) -> (queue out=w40:refnum<queue>, error out=w42:errorcluster)  [unwired: 3 in, 1 out]
  n10 = Enqueue Element(queue=w40, element="initialize", error in (no error)=w42) -> (queue out=w30:refnum<queue>, error out=w41:errorcluster)  [unwired: 1 in, 1 out]
  n11 = Bundle(cluster=T14 {"semaphore files"=refnum, "semaphore port"=refnum, "notifier read request"=refnum, "queue data"=refnum, "queue instructions"=refnum}, "semaphore files"=w13, "semaphore port"=w32, "notifier read request"=w31, "queue data"=w3, "queue instructions"=w30) -> (w6:T14)
  n12 = Unbundle By Name(w6) -> ("queue instructions"=w9:refnum<queue>)
  n13 = Unbundle By Name(w6) -> ("notifier read request"=w11:refnum<notifier>)
  n14 = Unbundle By Name(w6) -> ("queue instructions"=w20:refnum<queue>, "semaphore port"=w19:T13, "semaphore files"=w18:T13)
  n15 = Unbundle By Name(w6) -> ("queue data"=w17:refnum<queue>, "semaphore port"=w16:T13, "notifier read request"=w15:refnum<notifier>)
  n16 = Unbundle By Name(w6) -> ("semaphore files"=w12:T13)
  n17 = Unbundle By Name(w6) -> ("semaphore files"=w5:T13)
  n18 = Unbundle By Name(w6) -> ("queue data"=w14:refnum<queue>)
  n19 = while {
    shift-right: [w53] -> w21
    shift-left: w41 -> [w56]
    tunnel: w11 -> [w50]
    tunnel: w9 -> [w49]
    tunnel: w5 -> [w48]
    stop <- w54 stop-if-true
    # "producer loop"
    n20 = event shown="[18] \"settings 2ch\": Value Change" {
      selector: _ -> [_ _ _ _ _ _ _ _ _ _ _ _ _ _ _ _ _ _ _ _]
      dyn-events: _ -> [_ _ _ _ _ _ _ _ _ _ _ _ _ _ _ _ _ _ _ _]
      timeout: 5 ("Numeric") -> [_ _ _ _ _ _ _ _ _ _ _ _ _ _ _ _ _ _ _ _]
      tunnel: w49 -> [w63 w90 w155 w167 w175 w195 w198 w206 w209 w216 _ w226 w259 w306 w310 w319 w327 w335 _ _]
      tunnel: w56 -> [w64 w89 w156 w169 w178 w196 w200 w207 w211 w214 w223 w228 w272 w304 w308 w312 w320 w328 w337 w344]
      tunnel: [w62 w88 w154 w168 w180 w192 w199 w204 w210 w215 w222 w227 w260 w305 w309 w318 w326 w334 w336 w344] -> w53
      tunnel: [w57 _ _ _ _ _ _ _ _ _ _ _ _ _ _ _ _ _ _ _] -> w55
      tunnel: w50 -> [_ w91 _ _ _ _ _ _ _ _ _ _ _ _ _ _ _ _ _ _]
      tunnel: w48 -> [_ _ _ _ _ _ _ _ _ _ _ _ w273 _ _ _ _ _ _ _]
      event "butExit": Value Change {
        n21 = event-data() -> ()  [unwired: 1 in, 1 out]
        n22 = Two Button Dialog(message="Are you sure you want to exit the program?", 1:"No" ("F button name (\"Cancel\")"), 2:"Yes" ("T button name (\"OK\")")) -> (T button?=w57:bool)
        n23 = case shown="True" w57 {
          tunnel: w64 -> [w65 w73]
          tunnel: w63 -> [_ w72]
          tunnel: [w65 w66] -> w62
          frame False {
          }
          frame True {
            n24 = Enqueue Element(queue=w72, element="disconnect", error in (no error)=w73) -> (queue out=w70:refnum<queue>, error out=w71:errorcluster)  [unwired: 1 in, 1 out]
            n25 = Enqueue Element(queue=w70, element="close program", error in (no error)=w71) -> (queue out=w67:refnum<queue>, error out=w68:errorcluster)  [unwired: 1 in, 1 out]
            n26 = while "waits 5s for queue to empty" {
              shift-right: [w83] -> w66
              shift-left: w68 -> [w85]
              shift-right: [w80] -> _
              shift-left: w67 -> [w84]
              i -> [w79]
              stop <- w75 stop-if-true
              n27 = Greater?(x=w79, y=50) -> (0:w76:bool)
              n28 = Get Queue Status(queue=w84, error in (no error)=w85) -> (queue out=w80:refnum<queue>, error out=w83:errorcluster, # elements in queue=w82:i32)  [unwired: 1 in, 5 out]
              n29 = Greater Than 0?(x=w82) -> (x > 0?=w77:bool)
              n30 = Wait (ms)(milliseconds to wait=u32 100 ("refresh rate")) -> ()  [unwired: 1 out]
              n31 = Or(x=w77, y=w76) -> (x .or. y?=w75:bool)
            }
          }
        }
        n32 = local write "butExit"(FALSE ("butStop")) -> ()
      }
      event Timeout {
        n33 = event-data() -> ()  [unwired: 1 in, 1 out]
        n34 = Get Date/Time In Seconds() -> (seconds since 1Jan1904=w87:timestamp)
        "timer-current" <- w87
        n35 = local read "connection state"() -> (w86:T8)
        n36 = case shown="\"acquiring data\"" w86 {
          tunnel: w89 -> [w92 w94 w114 w140]
          tunnel: w90 -> [_ w95 w117 w139]
          tunnel: [w92 w96 w118 w138] -> w88
          tunnel: w87 -> [_ w93 w111 w137]
          tunnel: w91 -> [_ _ w112 _]
          frame "disconnected", Default {
          }
          frame "connected" {
            n37 = local read "timer-settings"() -> (w99:timestamp)
            n38 = Get Queue Status(queue=w95, error in (no error)=w94) -> (queue out=w103:refnum<queue>, error out=w104:errorcluster, # elements in queue=w101:i32)  [unwired: 1 in, 5 out]
            n39 = Increment(x=w99) -> (x+1=w100:timestamp)
            n40 = Greater Or Equal?(x=w93, y=w100) -> (x >= y?=w97:bool)
            n41 = Equal To 0?(x=w101) -> (x = 0?=w98:bool)
            n42 = And(x=w98, y=w97) -> (x .and. y?=w102:bool)
            n43 = case "if empty queue &\ntime to read settings" shown="True" w102 {
              tunnel: w104 -> [w105 w110]
              tunnel: [w105 w109] -> w96
              tunnel: w103 -> [_ w108]
              tunnel: w93 -> [_ w106]
              frame False {
              }
              frame True {
                n44 = local write "timer-settings"(w106) -> ()
                n45 = Enqueue Element(queue=w108, element="get settings", error in (no error)=w110) -> (error out=w109:errorcluster)  [unwired: 1 in, 2 out]
              }
            }
          }
          frame "acquiring data" {
            n46 = local read "timer-nextRead"() -> (w116:timestamp)
            n47 = local read "timer-settings"() -> (w121:timestamp)
            n48 = Greater Or Equal?(x=w111, y=w116) -> (x >= y?=w115:bool)
            n49 = case "if time to read samples" shown="True" w115 {
              tunnel: [w127 w131] -> w113
              tunnel: w114 -> [w127 w130]
              tunnel: w112 -> [_ w129]
              tunnel: w111 -> [_ w128]
              frame False {
              }
              frame True {
                n50 = Send Notification(notification=w128, notifier=w129, error in (no error)=w130) -> (error out=w131:errorcluster)  [unwired: 1 out]
              }
            }
            n51 = Increment(x=w121) -> (x+1=w122:timestamp)
            n52 = Greater Or Equal?(x=w111, y=w122) -> (x >= y?=w119:bool)
            n53 = Get Queue Status(queue=w117, error in (no error)=w113) -> (queue out=w125:refnum<queue>, error out=w126:errorcluster, # elements in queue=w123:i32)  [unwired: 1 in, 5 out]
            n54 = Equal To 0?(x=w123) -> (x = 0?=w120:bool)
            n55 = And(x=w120, y=w119) -> (x .and. y?=w124:bool)
            n56 = case "if empty queue &\ntime to read settings" shown="True" w124 {
              tunnel: w126 -> [w132 w136]
              tunnel: [w132 w135] -> w118
              tunnel: w125 -> [_ w134]
              frame False {
              }
              frame True {
                n57 = Enqueue Element(queue=w134, element="get settings", error in (no error)=w136) -> (error out=w135:errorcluster)  [unwired: 1 in, 2 out]
              }
            }
          }
          frame "connection error", "acquisition error" {
            n58 = local read "timer-reconnect"() -> (w146:timestamp)
            n59 = Get Queue Status(queue=w139, error in (no error)=w140) -> (queue out=w142:refnum<queue>, error out=w141:errorcluster, # elements in queue=w144:i32)  [unwired: 1 in, 5 out]
            n60 = Increment(x=w146) -> (x+1=w145:timestamp)
            n61 = Equal To 0?(x=w144) -> (x = 0?=w147:bool)
            n62 = Greater Or Equal?(x=w137, y=w145) -> (x >= y?=w148:bool)
            n63 = And(x=w147, y=w148) -> (x .and. y?=w143:bool)
            n64 = case "if empty queue & time to try reconnection" shown="True" w143 {
              tunnel: w141 -> [w149 w153]
              tunnel: [w149 w152] -> w138
              tunnel: w142 -> [_ w151]
              frame False {
              }
              frame True {
                n65 = Enqueue Element(queue=w151, element="reconnect", error in (no error)=w153) -> (error out=w152:errorcluster)  [unwired: 1 in, 2 out]
              }
            }
          }
        }
      }
      event "butConnect": Value Change {
        n66 = event-data() -> ()  [unwired: 1 in, 1 out]
        n67 = Enqueue Element(queue=w155, element="connect", error in (no error)=w156) -> (error out=w154:errorcluster)  [unwired: 1 in, 2 out]
      }
      event "butDisconnect": Value Change {
        n68 = event-data() -> ()  [unwired: 1 in, 1 out]
        n69 = local read "connection state"() -> (w165:T8)
        n70 = Equal?(x=connectionState."connection error" ("connection state"), y=w165) -> (x = y?=w162:bool)
        n71 = Equal?(x=w165, y=connectionState."acquisition error" ("connection state")) -> (x = y?=w163:bool)
        n72 = Or(x=w162, y=w163) -> (x .or. y?=w161:bool)
        n73 = Select(t="disconnect when error" ("element"), s=w161, f="disconnect" ("element")) -> (s? t:f=w158:string)
        n74 = Enqueue Element(queue=w167, element=w158, error in (no error)=w169) -> (error out=w168:errorcluster)  [unwired: 1 in, 2 out]
      }
      event "butStartAcq": Value Change {
        n75 = event-data() -> ()  [unwired: 1 in, 1 out]
        n76 = local read "dataTable"() -> (w171:string[][])
        n77 = Enqueue Element(queue=w175, element="lock settings", error in (no error)=w178) -> (queue out=w174:refnum<queue>, error out=w177:errorcluster)  [unwired: 1 in, 1 out]
        n78 = Empty Array?(array=w171) -> (empty?=w170:bool)
        n79 = Enqueue Element(queue=w174, element="reset timers", error in (no error)=w177) -> (queue out=w182:refnum<queue>, error out=w183:errorcluster)  [unwired: 1 in, 1 out]
        n80 = case shown="True" w170 {
          tunnel: w183 -> [w185 w190]
          tunnel: w182 -> [w184 w189]
          tunnel: [w185 w188] -> w181
          tunnel: [w184 w187] -> w179
          frame False {
          }
          frame True {
            n81 = Enqueue Element(queue=w189, element="create file", error in (no error)=w190) -> (queue out=w187:refnum<queue>, error out=w188:errorcluster)  [unwired: 1 in, 1 out]
          }
        }
        n82 = Enqueue Element(queue=w179, element="start acquisition", error in (no error)=w181) -> (error out=w180:errorcluster)  [unwired: 1 in, 2 out]
      }
      event "butStopAcq": Value Change {
        n83 = event-data() -> ()  [unwired: 1 in, 1 out]
        n84 = Enqueue Element(queue=w195, element="stop acquisition", error in (no error)=w196) -> (queue out=w191:refnum<queue>, error out=w193:errorcluster)  [unwired: 1 in, 1 out]
        n85 = Enqueue Element(queue=w191, element="unlock settings", error in (no error)=w193) -> (error out=w192:errorcluster)  [unwired: 1 in, 2 out]
      }
      event "butUnlockSett": Value Change {
        n86 = event-data() -> ()  [unwired: 1 in, 1 out]
        n87 = Enqueue Element(queue=w198, element="unlock settings", error in (no error)=w200) -> (error out=w199:errorcluster)  [unwired: 1 in, 2 out]
      }
      event "butLoadDefSett": Value Change {
        n88 = event-data() -> ()  [unwired: 1 in, 1 out]
        n89 = Enqueue Element(queue=w206, element="set default settings", error in (no error)=w207) -> (queue out=w202:refnum<queue>, error out=w205:errorcluster)  [unwired: 1 in, 1 out]
        n90 = Enqueue Element(queue=w202, element="get settings", error in (no error)=w205) -> (error out=w204:errorcluster)  [unwired: 1 in, 2 out]
      }
      event "path-file": Key Down; "path-file": Mouse Down {
        n91 = event-data() -> ()  [unwired: 1 in, 1 out]
        n92 = Enqueue Element(queue=w209, element="get new filepath", error in (no error)=w211) -> (error out=w210:errorcluster)  [unwired: 1 in, 2 out]
      }
      event "error": Value Change {
        n93 = event-data() -> ("NewVal"=w213:errorcluster)  [unwired: 1 in]
        n94 = case shown="Error" w213 {
          tunnel: w214 -> [w217 w220]
          tunnel: w216 -> [_ w219]
          tunnel: [w217 w218] -> w215
          frame No Error {
          }
          frame Error {
            n95 = Enqueue Element(queue=w219, element="handle error", error in (no error)=w220) -> (error out=w218:errorcluster)  [unwired: 1 in, 2 out]
          }
        }
      }
      event Panel Close? {
        n96 = event-data() -> ()  [unwired: 1 in, 4 out]
        n97 = property on="butExit" class="Bool (strict)"(error in=w223, "Val(Sgnl)"=TRUE ("Value (Signaling)")) -> (error out=w222:errorcluster)  [unwired: 1 in, 1 out]
        n98 = event-data("Discard?"=TRUE) -> ()  [unwired: 1 in, 1 out]
      }
      event Menu Selection (User) {
        n99 = event-data() -> ("ItemTag"=w229:string)  [unwired: 1 in]
        n100 = case shown="\"Default settings\"" w229 {
          tunnel: w228 -> [w230 w232 w237 w248 w250]
          tunnel: [w230 w231 w236 w247 w249] -> w227
          tunnel: w226 -> [_ _ _ w245 _]
          frame Default {
          }
          frame "Exit" {
            n101 = property on="butExit" class="Bool (strict)"(error in=w232, "Val(Sgnl)"=TRUE ("Value (Signaling)")) -> (error out=w231:errorcluster)  [unwired: 1 in, 1 out]
          }
          frame "Default settings" {
            w242 = 128  # call and forget
            n102 = vi-ref <instrlib>:"defaultSettingsDialog.vi"() -> (w241:refnum<vi>)
            n103 = local read "path-defsettings"() -> (w235:path)
            n104 = property class="VI"(reference=w241, error in=w237) -> (error out=w244:errorcluster, "Name"=w243:string)  [unwired: 1 out]
            n105 = control-ref of="default settings"() -> (w234:refnum<vi>)
            n106 = Open VI Reference(type specifier VI Refnum (for type only)=refnum<vi> refnum, vi path=w243, options=w242, error in (no error)=w244) -> (vi reference=w239:refnum<vi>, error out=w238:errorcluster)  [unwired: 2 in]
            n107 = call-by-ref "Start Asynchronous Call"(reference=w239, error in=w238, "default settings ref"=w234, "default settings path"=w235) -> (error out=w236:errorcluster)  [unwired: 9 in, 2 out]
          }
          frame "Save as" {
            n108 = Enqueue Element(queue=w245, element="get new filepath", error in (no error)=w248) -> (error out=w247:errorcluster)  [unwired: 1 in, 2 out]
          }
          frame "About" {
            w255 = 128  # call and forget
            n109 = vi-ref <instrlib>:"aboutDialog.vi"() -> (w254:refnum<vi>)
            n110 = property class="VI"(reference=w254, error in=w250) -> (error out=w257:errorcluster, "Name"=w256:string)  [unwired: 1 out]
            n111 = Open VI Reference(type specifier VI Refnum (for type only)=refnum<vi> refnum, vi path=w256, options=w255, error in (no error)=w257) -> (vi reference=w252:refnum<vi>, error out=w251:errorcluster)  [unwired: 2 in]
            n112 = call-by-ref "Start Asynchronous Call"(reference=w252, error in=w251) -> (error out=w249:errorcluster)  [unwired: 11 in, 2 out]
          }
        }
      }
      event Value Change {
        n113 = event-data() -> ("OldVal"=w266:T7, "NewVal"=w264:T7)  [unwired: 1 in]
        n114 = local read "path-settings"() -> (w281:path)
        n115 = local read "path-file"() -> (w275:path)
        n116 = call <instrlib>:"buildDefaultPath.vi"("default settings"=w264) -> ("settings path"=w282:path, "data path"=w271:path)  [unwired: 3 in]
        n117 = call <vilib>:"Acquire Semaphore.vi"("error in (no error)"=w272, "semaphore"=w273) -> ("error out"=w276:errorcluster, "semaphore out"=w278:T13)  [unwired: 3 in, 1 out]
        n118 = Not Equal?(x=w275, y=w271) -> (x != y?=w280:bool)
        n119 = Not Equal?(x=w282, y=w281) -> (x != y?=w279:bool)
        n120 = Or(x=w280, y=w279) -> (x .or. y?=w274:bool)
        n121 = case "path changed?" shown="True" w274 {
          tunnel: w259 -> [w296 w302]
          tunnel: w276 -> [w297 w301]
          tunnel: w271 -> [_ w299]
          tunnel: [w297 w300] -> w277
          tunnel: [w296 w298] -> w258
          frame False {
          }
          frame True {
            n122 = local write "path-new"(w299) -> ()
            n123 = Enqueue Element(queue=w302, element="rename files", error in (no error)=w301) -> (queue out=w298:refnum<queue>, error out=w300:errorcluster)  [unwired: 1 in, 1 out]
          }
        }
        n124 = Unbundle By Name(w266) -> ("delimiter"=w268:string)
        n125 = Unbundle By Name(w264) -> ("delimiter"=w267:string)
        n126 = Unbundle By Name(w266) -> ("Abacus settings"=w265:T4)
        n127 = Unbundle By Name(w264) -> ("Abacus settings"=w263:T4)
        n128 = Not Equal?(x=w268, y=w267) -> (x != y?=w270:bool)
        n129 = call <vilib>:"Release Semaphore.vi"("error in (no error)"=w277, "semaphore"=w278) -> ("error out"=w269:errorcluster)  [unwired: 4 in, 1 out]
        n130 = case "delimiter changed?" shown="True" w270 {
          tunnel: [w290 w294] -> w261
          tunnel: w258 -> [w289 w293]
          tunnel: w269 -> [w290 w292]
          tunnel: [w289 w291] -> w262
          frame False {
          }
          frame True {
            n131 = Enqueue Element(queue=w293, element="edit file delimiter", error in (no error)=w292) -> (queue out=w291:refnum<queue>, error out=w294:errorcluster)  [unwired: 1 in, 1 out]
          }
        }
        n132 = Not Equal?(x=w265, y=w263) -> (x != y?=w283:bool)
        n133 = case "def. settings changed?" shown="True" w283 {
          tunnel: w262 -> [_ w287]
          tunnel: w261 -> [w284 w286]
          tunnel: [w284 w285] -> w260
          frame False {
          }
          frame True {
            n134 = Enqueue Element(queue=w287, element="set default settings", error in (no error)=w286) -> (error out=w285:errorcluster)  [unwired: 1 in, 2 out]
          }
        }
      }
      event Value Change {
        n135 = event-data() -> ()  [unwired: 1 in, 2 out]
        n136 = Enqueue Element(queue=w306, element="set sampling", error in (no error)=w304) -> (error out=w305:errorcluster)  [unwired: 1 in, 2 out]
      }
      event Value Change {
        n137 = event-data() -> ()  [unwired: 1 in, 2 out]
        n138 = Enqueue Element(queue=w310, element="set coincidence window", error in (no error)=w308) -> (error out=w309:errorcluster)  [unwired: 1 in, 2 out]
      }
      event Value Change {
        n139 = event-data() -> ("CtlRef"=w317:refnum<vi>)  [unwired: 1 in, 2 out]
        n140 = property class="DigNum (strict)"(reference=w317) -> ("Label.Text"=w314:string)  [unwired: 1 in, 2 out]
        n141 = call <instrlib>:"getLastChar.vi"("string"=w314) -> ("last char"=w313:string)
        n142 = Concatenate Strings("set delay " ("element"), w313) -> (w315:string)
        n143 = Enqueue Element(queue=w319, element=w315, error in (no error)=w312) -> (error out=w318:errorcluster)  [unwired: 1 in, 2 out]
      }
      event Value Change {
        n144 = event-data() -> ("CtlRef"=w325:refnum<vi>)  [unwired: 1 in, 2 out]
        n145 = property class="DigNum (strict)"(reference=w325) -> ("Label.Text"=w322:string)  [unwired: 1 in, 2 out]
        n146 = call <instrlib>:"getLastChar.vi"("string"=w322) -> ("last char"=w321:string)
        n147 = Concatenate Strings("set sleep " ("element"), w321) -> (w323:string)
        n148 = Enqueue Element(queue=w327, element=w323, error in (no error)=w320) -> (error out=w326:errorcluster)  [unwired: 1 in, 2 out]
      }
      event Value Change {
        n149 = event-data() -> ("CtlRef"=w330:refnum<vi>)  [unwired: 1 in, 2 out]
        n150 = property class="Ring (strict)"(reference=w330) -> ("Label.Text"=w332:string)  [unwired: 1 in, 2 out]
        n151 = call <instrlib>:"getLastChar.vi"("string"=w332) -> ("last char"=w331:string)
        n152 = Concatenate Strings("set multi " ("element"), w331) -> (w329:string)
        n153 = Enqueue Element(queue=w335, element=w329, error in (no error)=w328) -> (error out=w334:errorcluster)  [unwired: 1 in, 2 out]
      }
      event Value Change {
        n154 = event-data() -> ()  [unwired: 1 in, 6 out]
        n155 = call <instrlib>:"Settings2ch To Settings4ch.vi"("settings2ch"="settings 2ch") -> ("settings4ch"=w338:T4)
        n156 = property on="settings 4ch" class="Clust (strict)"(error in=w337, "Val(Sgnl)"=w338) -> (error out=w336:errorcluster)  [unwired: 1 in, 1 out]
      }
      event Value Change {
        n157 = event-data() -> ("OldVal"=w343:T4, "NewVal"=w342:T4)  [unwired: 1 in, 4 out]
        n158 = Not Equal?(x=w343, y=w342) -> (x != y?=w341:T16)
        n159 = Cluster To Array(cluster=w341) -> (array=→"sttgs changed?":bool[])
      }
    }
    n160 = Unbundle By Name(w53) -> ("status"=w52:bool)
    n161 = Or(x=w52, y=w55) -> (x .or. y?=w54:bool)
  }
  n162 = while {
    tunnel: w20 -> [w345]
    tunnel: w19 -> [w348]
    tunnel: w18 -> [w347]
    stop <- w349 stop-if-true
    # "instruction consumer loop"
    n163 = Dequeue Element(queue=w345) -> (queue out=w346:refnum<queue>, element=w350:string, error out=w351:errorcluster)  [unwired: 2 in, 1 out]
    n164 = case shown="No Error" w351 {
      selector: w351 -> [w352 _]
      tunnel: w350 -> [w356 _]
      tunnel: [_ TRUE] -> w349
      tunnel: w348 -> [w355 _]
      tunnel: w347 -> [w354 _]
      tunnel: w346 -> [w353 _]
      frame No Error {
        n165 = case shown="\"reset values\"" w356 {
          selector: w356 -> [_ _ _ _ _ _ _ _ _ _ _ _ _ _ _ _ _ _ _ _ _ _ w908 w963 _ _ w1042 _ _ _ _]
          tunnel: w355 -> [_ w372 _ _ w451 _ _ w496 _ w561 _ _ _ w662 w695 _ _ _ _ _ w843 w853 w907 w964 w1004 _ w1041 _ _ _ _]
          tunnel: w354 -> [w361 w371 w417 w421 w442 _ w473 w495 w539 w560 w597 _ _ _ w679 w744 _ _ _ _ w834 w852 w898 w954 w996 _ w1032 w1083 w1102 _ _]
          tunnel: w353 -> [_ w368 _ _ _ _ _ _ w546 _ w616 w650 _ w660 w690 _ _ _ _ _ _ _ _ _ _ w1013 _ _ _ _ _]
          tunnel: w352 -> [_ _ _ _ _ _ _ w494 w538 w559 w614 w649 _ _ _ _ _ _ _ _ _ w854 _ _ _ w1012 _ _ _ _ _]
          frame "close program" {
            n166 = local read "dataTable"() -> (w360:string[][])
            n167 = Empty Array?(array=w360) -> (empty?=w359:bool)
            n168 = case shown="True" w359 {
              tunnel: w361 -> [_ w367]
              frame False {
              }
              frame True {
                # "if no data taken, delete settings file"
                n169 = call <vilib>:"Acquire Semaphore.vi"("semaphore"=w367) -> ("error out"=w365:errorcluster, "semaphore out"=w366:T13)  [unwired: 4 in, 1 out]
                n170 = property on="path-settings" class="Path"(error in=w365) -> (error out=w363:errorcluster, "Value"=w364:path)  [unwired: 1 in, 1 out]
                n171 = Delete(path (use dialog)=w364, error in=w363) -> (error out=w362:errorcluster)  [unwired: 3 in, 2 out]
                n172 = call <vilib>:"Release Semaphore.vi"("error in (no error)"=w362, "semaphore"=w366) -> ()  [unwired: 4 in, 2 out]
              }
            }
            n173 = call <instrlib>:"prependTimestamp.vi"("string in"="Closing program" ("status str")) -> ("string out"=w357:string)  [unwired: 14 in]
            n174 = local write "status"(w357) -> ()
          }
          frame "connect" {
            n175 = call <instrlib>:"connectToDevice.vi"() -> ("selected device type"=w370:T6, "selected VISA"=w369:refnum<visa-resource-name>, "Cancelled?"=w374:bool)  [unwired: 8 in, 1 out]
            "device type" <- w370
            n176 = Not(x=w374) -> (.not. x?=w373:bool)
            n177 = case shown="True" w373 {
              tunnel: w372 -> [_ w380]
              tunnel: w371 -> [_ w379]
              tunnel: w370 -> [_ w378]
              tunnel: w369 -> [_ w377]
              tunnel: w368 -> [_ w376]
              frame False {
                n178 = local write "connection state"(connectionState."disconnected" ("connection state")) -> ()
              }
              frame True {
                n179 = stacked-sequence {
                  tunnel: w380 -> [w383 _ _]
                  tunnel: w379 -> [_ w394 _]
                  tunnel: w378 -> [_ w391 w402]
                  tunnel: w377 -> [w382 w392 _]
                  tunnel: w376 -> [w381 _ _]
                  frame #0 {
                    n180 = call <vilib>:"Acquire Semaphore.vi"("semaphore"=w383) -> ("error out"=w385:errorcluster, "semaphore out"=w386:T13)  [unwired: 4 in, 1 out]
                    n181 = call <instrlib>:"Open.vi"("error in (no error)"=w385, "VISA resource name"=w382) -> ("error out"=w384:errorcluster, "VISA resource name out"=→"abacus VISA":refnum<visa-resource-name>)  [unwired: 8 in]
                    n182 = call <vilib>:"Release Semaphore.vi"("error in (no error)"=w384, "semaphore"=w386) -> ("error out"=w388:errorcluster)  [unwired: 4 in, 1 out]
                    n183 = Enqueue Element(queue=w381, element="get initial settings", error in (no error)=w388) -> ()  [unwired: 1 in, 3 out]
                  }
                  frame #1 {
                    n184 = call <instrlib>:"connectionStatusString.vi"("connected? [T]"=TRUE, "device type"=w391, "Abacus VISA"=w392) -> ("String"=w393:string)  [unwired: 8 in]
                    n185 = call <vilib>:"Acquire Semaphore.vi"("semaphore"=w394) -> ("error out"=w398:errorcluster, "semaphore out"=w396:T13)  [unwired: 4 in, 1 out]
                    n186 = local read "delimiter"() -> (w400:string)
                    n187 = property on="path-settings" class="Path"(error in=w398) -> (error out=w399:errorcluster, "Value"=w397:path)  [unwired: 1 in, 1 out]
                    n188 = call <instrlib>:"writeSettingsFile4ch.vi"("delimiter (,)"=w400, "message (overrides settings)"=w393, "error in (no error)"=w399, "path"=w397) -> ("error out"=w401:errorcluster)  [unwired: 6 in, 1 out]
                    n189 = call <instrlib>:"prependTimestamp.vi"("string in"=w393) -> ("string out"=w395:string)  [unwired: 14 in]
                    n190 = call <vilib>:"Release Semaphore.vi"("error in (no error)"=w401, "semaphore"=w396) -> ()  [unwired: 4 in, 2 out]
                    n191 = local write "status"(w395) -> ()
                  }
                  frame #2 {
                    w403 = connectionState."connected" ("connection state")
                    n192 = local read "ref indics"() -> (w405:T2)
                    n193 = local read "ref ctrls"() -> (w404:T1)
                    n194 = local write "connection state"(w403) -> ()
                    n195 = call <instrlib>:"controlVisibility4Ch.vi"("device type [AB1004]"=w402, "ref controls"=w404, "connection state"=w403) -> ()  [unwired: 9 in]
                    n196 = call <instrlib>:"indicatorVisibility4Ch.vi"("device type [AB1004]"=w402, "ref indics"=w405) -> ()  [unwired: 10 in]
                  }
                }
              }
            }
          }
          frame "create file" {
            # "Clears the file if it exists, creates it if is new."
            n197 = local read "device type"() -> (w407:T6)
            n198 = case shown="1004, 1504, 1904, 2004, 2504, Default" w407 {
              tunnel: [string[] ["Time (s)", "Data ID", "Counts A", "Counts B", "Counts C", "Counts D", "Coincidences AB", "Coincidences AC", "Coincidences AD", "Coincidences BC", "Coincidences BD", "Coincidences CD", "Multi-fold"] string[] ["Time (s)", "Data ID", "Counts A", "Counts B", "Coincidences AB"]] -> w406
              frame 1004, 1504, 1904, 2004, 2504, Default {
              }
              frame 1002, 1502, 1902 {
              }
            }
            "dafafile header" <- w406
            n199 = call <vilib>:"Acquire Semaphore.vi"("semaphore"=w417) -> ("error out"=w411:errorcluster, "semaphore out"=w416:T13)  [unwired: 4 in, 1 out]
            n200 = local read "delimiter"() -> (w408:string)
            n201 = property on="path-file" class="Path"(error in=w411) -> (error out=w410:errorcluster, "Value"=w409:path)  [unwired: 1 in, 1 out]
            n202 = call-poly <vilib>:"Write Delimited Spreadsheet.vi"("file path (dialog if empty)"=w409, "1D data"=w406, "append to file? (F)"=FALSE, "error in (no error)"=w410, "delimiter (\\t)"=w408) -> ("new file path (Not A Path if cancelled)"=w414:path, "error out"=w413:errorcluster)  [unwired: 9 in]
            n203 = property on="path-file" class="Path"(error in=w413, "Value"=w414) -> (error out=w412:errorcluster)  [unwired: 1 in, 1 out]
            n204 = call <vilib>:"Release Semaphore.vi"("error in (no error)"=w412, "semaphore"=w416) -> ()  [unwired: 4 in, 2 out]
          }
          frame "create settings file" {
            n205 = local read "timer-begin"() -> (w428:timestamp)
            n206 = Format Date/Time String(time format string (%c)="%Y/%m/%d %H:%M:%S", seconds (now)=w428) -> (date/time string=w426:string)  [unwired: 1 in]
            n207 = call <vilib>:"Space Constant.vi"() -> ("String"=w429:string)
            n208 = Concatenate Strings("##### SETTINGS FILE #####\nTausand Abacus session began at", w429, w426) -> (w433:string)
            n209 = call <vilib>:"Acquire Semaphore.vi"("semaphore"=w421) -> ("error out"=w425:errorcluster, "semaphore out"=w424:T13)  [unwired: 4 in, 1 out]
            n210 = Build Array(w433) -> (w432:string[])
            n211 = property on="path-settings" class="Path"(error in=w425) -> (error out=w422:errorcluster, "Value"=w423:path)  [unwired: 1 in, 1 out]
            n212 = call-poly <vilib>:"Write Delimited Spreadsheet.vi"("file path (dialog if empty)"=w423, "1D data"=w432, "append to file? (F)"=FALSE, "error in (no error)"=w422) -> ("error out"=w420:errorcluster)  [unwired: 10 in, 1 out]
            n213 = call <vilib>:"Release Semaphore.vi"("error in (no error)"=w420, "semaphore"=w424) -> ()  [unwired: 4 in, 2 out]
          }
          frame "disconnect" {
            n214 = local read "abacus VISA"() -> (w436:refnum<visa-resource-name>)
            n215 = call <vilib>:"Acquire Semaphore.vi"("semaphore"=w451) -> ("error out"=w446:errorcluster, "semaphore out"=w447:T13)  [unwired: 4 in, 1 out]
            n216 = local read "device type"() -> (w435:T6)
            n217 = call <instrlib>:"Close.vi"("error in (no error)"=w446, "VISA resource name"=w436) -> ("error out"=w445:errorcluster)  [unwired: 9 in]
            n218 = call <vilib>:"Release Semaphore.vi"("error in (no error)"=w445, "semaphore"=w447) -> ()  [unwired: 4 in, 2 out]
            n219 = call <instrlib>:"connectionStatusString.vi"("connected? [T]"=FALSE, "device type"=w435, "Abacus VISA"=w436) -> ("String"=w437:string)  [unwired: 8 in]
            n220 = call <vilib>:"Acquire Semaphore.vi"("semaphore"=w442) -> ("error out"=w444:errorcluster, "semaphore out"=w443:T13)  [unwired: 4 in, 1 out]
            n221 = local read "delimiter"() -> (w438:string)
            n222 = property on="path-settings" class="Path"(error in=w444) -> (error out=w441:errorcluster, "Value"=w439:path)  [unwired: 1 in, 1 out]
            n223 = local read "connection state"() -> (w448:T8)
            n224 = call <instrlib>:"writeSettingsFile4ch.vi"("delimiter (,)"=w438, "message (overrides settings)"=w437, "error in (no error)"=w441, "path"=w439) -> ("error out"=w440:errorcluster)  [unwired: 6 in, 1 out]
            n225 = call <vilib>:"Release Semaphore.vi"("error in (no error)"=w440, "semaphore"=w443) -> ()  [unwired: 4 in, 2 out]
            n226 = case shown="\"connected\", Default" w448 {
              selector: w448 -> [_ w455 w456]
              tunnel: [connectionState."disconnected" ("connection state") w455 w456] -> w450
              tunnel: w437 -> [w452 _ _]
              frame "connected", Default {
                n227 = call <instrlib>:"prependTimestamp.vi"("string in"=w452) -> ("string out"=w453:string)  [unwired: 14 in]
                n228 = local write "status"(w453) -> ()
              }
              frame "connection error" {
              }
              frame "acquisition error" {
              }
            }
            n229 = local read "ref ctrls"() -> (w449:T1)
            n230 = local write "connection state"(w450) -> ()
            n231 = call <instrlib>:"controlVisibility4Ch.vi"("device type [AB1004]"=w435, "ref controls"=w449, "connection state"=w450) -> ()  [unwired: 9 in]
          }
          frame "disconnect when error" {
            w460 = connectionState."disconnected" ("connection state")
            n232 = local read "device type"() -> (w457:T6)
            n233 = local read "ref ctrls"() -> (w459:T1)
            n234 = property on="status" class="Str"("Text.TextColor"=u32 0) -> ()  [unwired: 2 in, 2 out]
            n235 = local write "connection state"(w460) -> ()
            n236 = call <instrlib>:"controlVisibility4Ch.vi"("device type [AB1004]"=w457, "ref controls"=w459, "connection state"=w460) -> ()  [unwired: 9 in]
          }
          frame "edit file delimiter" {
            n237 = call <vilib>:"Acquire Semaphore.vi"("semaphore"=w473) -> ("error out"=w469:errorcluster, "semaphore out"=w471:T13)  [unwired: 4 in, 1 out]
            n238 = local read "path-settings"() -> (w467:path)
            n239 = local read "default settings"() -> (w472:T7)
            n240 = local read "path-file"() -> (w468:path)
            n241 = property on="delimiter" class="Str"(error in=w469) -> (error out=w463:errorcluster, "Value"=w470:string)  [unwired: 1 in, 1 out]
            n242 = Build Array(w468, w467) -> (w466:path[])
            n243 = Unbundle By Name(w472) -> ("delimiter"=w462:string)
            n244 = case shown="\",\", \";\", Default" w462 {
              selector: w462 -> [_ _ w476]
              tunnel: [w474 "\t" w476] -> w461
              frame "Space", "space" {
                n245 = call <vilib>:"Space Constant.vi"() -> ("String"=w474:string)
              }
              frame "Tab", "tab" {
              }
              frame ",", ";", Default {
              }
            }
            n246 = for {
              tunnel: w470 -> [w482]
              tunnel: w461 -> [w481]
              shift-right: [w479] -> w465
              shift-left: w463 -> [w480]
              tunnel: w466 -> [w478] mode=indexing
              n247 = call <vilib>:"Is Path and Not Empty.vi"("path"=w478) -> ("Is Path and Not Empty?"=w483:bool)  [unwired: 4 in]
              n248 = call <vilib>:"Check if File or Folder Exists.vi"("path"=w478) -> ("file or folder exists?"=w484:bool)  [unwired: 8 in, 2 out]
              n249 = And(x=w483, y=w484) -> (x .and. y?=w477:bool)
              n250 = case shown="True" w477 {
                tunnel: w482 -> [_ w493]
                tunnel: w481 -> [_ w492]
                tunnel: w480 -> [w485 w488]
                tunnel: [w485 w487] -> w479
                tunnel: w478 -> [_ w486]
                frame False {
                }
                frame True {
                  n251 = call-poly <vilib>:"Read Delimited Spreadsheet.vi"("file path (dialog if empty)"=w486, "error in (no error)"=w488, "delimiter (\\t)"=w493) -> ("new file path (Not A Path if cancelled)"=w490:path, "all rows"=w491:string[][], "error out"=w489:errorcluster)  [unwired: 7 in, 3 out]
                  n252 = call-poly <vilib>:"Write Delimited Spreadsheet.vi"("file path (dialog if empty)"=w490, "2D data"=w491, "error in (no error)"=w489, "delimiter (\\t)"=w492) -> ("error out"=w487:errorcluster)  [unwired: 10 in, 1 out]
                }
              }
            }
            n253 = property on="delimiter" class="Str"(error in=w465, "Value"=w461) -> (error out=w464:errorcluster)  [unwired: 1 in, 1 out]
            n254 = call <vilib>:"Release Semaphore.vi"("error in (no error)"=w464, "semaphore"=w471) -> ()  [unwired: 4 in, 2 out]
          }
          frame "get initial settings" {
            n255 = local read "connection state"() -> (w497:T8)
            n256 = case shown="\"connected\"" w497 {
              tunnel: w496 -> [_ w504]
              tunnel: w495 -> [_ w503]
              tunnel: w494 -> [_ w502]
              frame "disconnected", Default {
              }
              frame "connected" {
                # "fake old values to\nforce file writing"
                n257 = local read "abacus VISA"() -> (w507:refnum<visa-resource-name>)
                n258 = local read "device type"() -> (w513:T6)
                n259 = call <vilib>:"Acquire Semaphore.vi"("error in (no error)"=w502, "semaphore"=w504) -> ("error out"=w510:errorcluster, "semaphore out"=w505:T13)  [unwired: 3 in, 1 out]
                n260 = Initialize Array(u32 99999 ("delay_C"), 11 ("dimension size")) -> (w501:u32[])
                n261 = call <instrlib>:"Query All Settings.vi"("device type"=w513, "error in (no error)"=w510, "read timeout (500 ms)"=u32 250 ("read timeout (10000 ms)"), "VISA Refnum in"=w507) -> ("error out"=w508:errorcluster, "values"=w515:u32[], "labels"=w514:string[], "checksum ok?"=w511:bool)  [unwired: 3 in, 1 out]
                n262 = Array To Cluster(array=w501) -> (cluster=w498:T20)
                n263 = case shown="True" w511 {
                  tunnel: w498 -> [_ w530]
                  tunnel: w508 -> [w516 w518]
                  tunnel: [w516 w519] -> w509
                  tunnel: w514 -> [_ w532]
                  tunnel: w515 -> [_ w531]
                  tunnel: w503 -> [_ w517]
                  frame False {
                  }
                  frame True {
                    n264 = local read "settings 4ch"() -> (w520:T4)
                    n265 = local read "delimiter"() -> (w525:string)
                    n266 = call <instrlib>:"Bundle by Name Settings 4ch.vi"("input cluster settings 4ch"=w520, "names"=w532, "values"=w531) -> ("output cluster settings 4ch"=w521:T4)  [unwired: 12 in]
                    n267 = call <vilib>:"Acquire Semaphore.vi"("error in (no error)"=w518, "semaphore"=w517) -> ("error out"=w529:errorcluster, "semaphore out"=w523:T13)  [unwired: 3 in, 1 out]
                    n268 = property on="path-settings" class="Path"(error in=w529) -> (error out=w528:errorcluster, "Value"=w526:path)  [unwired: 1 in, 1 out]
                    n269 = call <instrlib>:"Settings4ch To Settings2ch.vi"("settings4ch"=w521) -> ("settings2ch"=w522:T3)
                    n270 = Get Date/Time In Seconds() -> (seconds since 1Jan1904=w524:timestamp)
                    "timer-settings 2" <- w524
                    n271 = local write "settings 2ch"(w522) -> ()
                    n272 = local write "settings_old"(w521) -> ()
                    n273 = local write "settings 4ch"(w521) -> ()
                    n274 = call <instrlib>:"writeSettingsFile4ch.vi"("delimiter (,)"=w525, "timestamp (current)"=w524, "error in (no error)"=w528, "old settings"=w530, "new settings"=w521, "path"=w526) -> ("error out"=w527:errorcluster)  [unwired: 4 in, 1 out]
                    n275 = call <vilib>:"Release Semaphore.vi"("error in (no error)"=w527, "semaphore"=w523) -> ("error out"=w519:errorcluster)  [unwired: 4 in, 1 out]
                  }
                }
                n276 = property on="error" class="Clust (strict)"("Val(Sgnl)"=w509) -> (error out=w506:errorcluster)  [unwired: 2 in, 1 out]
                n277 = call <vilib>:"Release Semaphore.vi"("error in (no error)"=w506, "semaphore"=w505) -> ()  [unwired: 4 in, 2 out]
              }
            }
          }
          frame "get new filepath" {
            n278 = local read "default settings"() -> (w535:T7)
            n279 = Unbundle By Name(w535) -> ("extension"=w536:string)
            n280 = local read "path-file"() -> (w543:path)
            n281 = case shown="\".csv\"" w536 {
              selector: w536 -> [_ w551]
              tunnel: ["Plain text data file" ("pattern label") "CSV (comma dellimited)" ("pattern label")] -> w534
              tunnel: [".dat" ("pattern (all files)") w551] -> w533
              frame ".dat", Default {
              }
              frame ".csv" {
              }
            }
            n282 = Strip Path(path=w543) -> (name=w547:string)  [unwired: 1 out]
            n283 = call "File Dialog"("start path"=w543, "prompt"="Save as... ", "default name"=w547, "error in"=w538, "pattern (all files)"=w533, "pattern label"=w534) -> ("selected path"=w544:path, "cancelled"=w545:bool, "error out"=w537:errorcluster)  [unwired: 6 in, 1 out]
            n284 = call <vilib>:"Acquire Semaphore.vi"("error in (no error)"=w537, "semaphore"=w539) -> ("error out"=w542:errorcluster, "semaphore out"=w540:T13)  [unwired: 3 in, 1 out]
            n285 = case shown="False" w545 {
              tunnel: w546 -> [w556 _]
              tunnel: w542 -> [w555 w558]
              tunnel: w544 -> [w553 _]
              tunnel: [w554 w558] -> w541
              frame False {
                n286 = Enqueue Element(queue=w556, element="rename files", error in (no error)=w555) -> (error out=w554:errorcluster)  [unwired: 1 in, 2 out]
                "path-new" <- w553
              }
              frame True {
              }
            }
            n287 = call <vilib>:"Release Semaphore.vi"("error in (no error)"=w541, "semaphore"=w540) -> ()  [unwired: 4 in, 2 out]
          }
          frame "get settings" {
            n288 = local read "connection state"() -> (w562:T8)
            n289 = case shown="\"connected\", \"acquiring data\"" w562 {
              tunnel: w561 -> [_ w565]
              tunnel: w560 -> [_ w564]
              tunnel: w559 -> [_ w563]
              frame "disconnected", Default {
              }
              frame "connected", "acquiring data" {
                n290 = local read "abacus VISA"() -> (w568:refnum<visa-resource-name>)
                n291 = local read "device type"() -> (w576:T6)
                n292 = property on="settings 4ch" class="Clust (strict)"(error in=w563) -> (error out=w574:errorcluster, "Value"=w575:T4)  [unwired: 1 in, 1 out]
                n293 = call <vilib>:"Acquire Semaphore.vi"("error in (no error)"=w574, "semaphore"=w565) -> ("error out"=w571:errorcluster, "semaphore out"=w566:T13)  [unwired: 3 in, 1 out]
                n294 = call <instrlib>:"Query All Settings.vi"("device type"=w576, "error in (no error)"=w571, "read timeout (500 ms)"=u32 250 ("read timeout (10000 ms)"), "VISA Refnum in"=w568) -> ("error out"=w569:errorcluster, "values"=w578:u32[], "labels"=w577:string[], "checksum ok?"=w572:bool)  [unwired: 3 in, 1 out]
                n295 = case shown="True" w572 {
                  tunnel: w575 -> [_ w593]
                  tunnel: w569 -> [w579 w581]
                  tunnel: [w579 w582] -> w570
                  tunnel: w577 -> [_ w595]
                  tunnel: w578 -> [_ w594]
                  tunnel: w564 -> [_ w580]
                  frame False {
                  }
                  frame True {
                    n296 = local read "settings 4ch"() -> (w583:T4)
                    n297 = local read "delimiter"() -> (w588:string)
                    n298 = call <instrlib>:"Bundle by Name Settings 4ch.vi"("input cluster settings 4ch"=w583, "names"=w595, "values"=w594) -> ("output cluster settings 4ch"=w584:T4)  [unwired: 12 in]
                    n299 = call <vilib>:"Acquire Semaphore.vi"("error in (no error)"=w581, "semaphore"=w580) -> ("error out"=w592:errorcluster, "semaphore out"=w586:T13)  [unwired: 3 in, 1 out]
                    n300 = property on="path-settings" class="Path"(error in=w592) -> (error out=w591:errorcluster, "Value"=w589:path)  [unwired: 1 in, 1 out]
                    n301 = call <instrlib>:"Settings4ch To Settings2ch.vi"("settings4ch"=w584) -> ("settings2ch"=w585:T3)
                    n302 = Get Date/Time In Seconds() -> (seconds since 1Jan1904=w587:timestamp)
                    "timer-settings" <- w587
                    n303 = local write "settings 2ch"(w585) -> ()
                    n304 = local write "settings_old"(w584) -> ()
                    n305 = local write "settings 4ch"(w584) -> ()
                    n306 = call <instrlib>:"writeSettingsFile4ch.vi"("delimiter (,)"=w588, "timestamp (current)"=w587, "error in (no error)"=w591, "old settings"=w593, "new settings"=w584, "path"=w589) -> ("error out"=w590:errorcluster)  [unwired: 4 in, 1 out]
                    n307 = call <vilib>:"Release Semaphore.vi"("error in (no error)"=w590, "semaphore"=w586) -> ("error out"=w582:errorcluster)  [unwired: 4 in, 1 out]
                  }
                }
                n308 = property on="error" class="Clust (strict)"("Val(Sgnl)"=w570) -> (error out=w567:errorcluster)  [unwired: 2 in, 1 out]
                n309 = call <vilib>:"Release Semaphore.vi"("error in (no error)"=w567, "semaphore"=w566) -> ()  [unwired: 4 in, 2 out]
              }
            }
          }
          frame "handle error" {
            n310 = Get Date/Time In Seconds() -> (seconds since 1Jan1904=w609:timestamp)
            n311 = local write "timer-reconnect"(w609) -> ()
            n312 = Flush Queue(queue=w616, error in (no error)=w614) -> (queue out=w615:refnum<queue>, error out=w613:errorcluster)  [unwired: 1 out]
            n313 = local read "error"() -> (w618:errorcluster)
            n314 = Enqueue Element(queue=w615, element="stop acquisition", error in (no error)=w613) -> (queue out=w605:refnum<queue>, error out=w604:errorcluster)  [unwired: 1 in, 1 out]
            n315 = Unbundle By Name(w618) -> ("code"=w617:i32, "source"=w611:string)
            n316 = Enqueue Element(queue=w605, element="disconnect", error in (no error)=w604) -> ()  [unwired: 1 in, 3 out]
            n317 = case shown="Default" w617 {
              tunnel: [w625 w629 w632] -> w603
              tunnel: [errorcluster {"status"=FALSE, "code"=0, "source"=""} ("no error constant") errorcluster {"status"=FALSE, "code"=0, "source"=""} ("no error constant") errorcluster {"status"=FALSE, "code"=0, "source"=""} ("no error constant")] -> w612
              tunnel: w611 -> [_ _ _]
              frame Default {
                w625 = "Connection lost." ("element")
                n318 = property on="status" class="Str"("Text.TextColor"=u32 16744448) -> ()  [unwired: 2 in, 2 out]
                n319 = call <instrlib>:"prependTimestamp.vi"("string in"=w625) -> ("string out"=→"status":string)  [unwired: 14 in]
              }
              frame 0 {
                n320 = disable-structure shown="Enabled" {
                  disable-tunnel: [w630 _] -> w629
                  frame Disabled {
                    w630 = "unknown error" ("message")
                    n321 = One Button Dialog(message=w630) -> ()  [unwired: 1 in, 1 out]
                  }
                  frame Enabled {
                    # "error code 0: unknown error source"
                  }
                }
              }
              frame -1073807360 {
                w632 = "Fatal Error. An error occurred at the communication port. Port is either closed or disconnected."
                n322 = One Button Dialog(message=w632) -> ()  [unwired: 1 in, 1 out]
              }
            }
            n323 = local read "connection state"() -> (w610:T8)
            n324 = case shown="\"connection error\"" w610 {
              selector: w610 -> [w619 _ _ w622 w623]
              tunnel: [w619 connectionState."connection error" ("connection state") connectionState."acquisition error" ("connection state") w622 w623] -> w608
              frame "disconnected", Default {
              }
              frame "connected" {
              }
              frame "acquiring data" {
              }
              frame "connection error" {
              }
              frame "acquisition error" {
              }
            }
            n325 = local write "error"(w612) -> ()
            n326 = call <vilib>:"Acquire Semaphore.vi"("semaphore"=w597) -> ("error out"=w602:errorcluster, "semaphore out"=w601:T13)  [unwired: 4 in, 1 out]
            n327 = local read "delimiter"() -> (w596:string)
            n328 = property on="path-settings" class="Path"(error in=w602) -> (error out=w599:errorcluster, "Value"=w598:path)  [unwired: 1 in, 1 out]
            n329 = local write "connection state"(w608) -> ()
            n330 = call <instrlib>:"writeSettingsFile4ch.vi"("delimiter (,)"=w596, "message (overrides settings)"=w603, "error in (no error)"=w599, "path"=w598) -> ("error out"=w600:errorcluster)  [unwired: 6 in, 1 out]
            n331 = call <vilib>:"Release Semaphore.vi"("error in (no error)"=w600, "semaphore"=w601) -> ()  [unwired: 4 in, 2 out]
          }
          frame "initialize" {
            n332 = disable-structure shown="RUN_TIME_ENGINE==True" {
              frame condition #0 (active) {
                n333 = property on="butExit" class="Bool (strict)"("Visible"=TRUE) -> ()  [unwired: 2 in, 2 out]
              }
              frame condition #1 {
                n334 = property on="butExit" class="Bool (strict)"("Visible"=FALSE) -> ()  [unwired: 2 in, 2 out]
              }
            }
            n335 = Enqueue Element(queue=w650, element="reset controls", error in (no error)=w649) -> (queue out=w634:refnum<queue>, error out=w637:errorcluster)  [unwired: 1 in, 1 out]
            n336 = Enqueue Element(queue=w634, element="reset indicators", error in (no error)=w637) -> (queue out=w635:refnum<queue>, error out=w636:errorcluster)  [unwired: 1 in, 1 out]
            n337 = Enqueue Element(queue=w635, element="reset values", error in (no error)=w636) -> (queue out=w646:refnum<queue>, error out=w647:errorcluster)  [unwired: 1 in, 1 out]
            n338 = Enqueue Element(queue=w646, element="reset timers", error in (no error)=w647) -> (queue out=w640:refnum<queue>, error out=w642:errorcluster)  [unwired: 1 in, 1 out]
            n339 = Enqueue Element(queue=w640, element="create settings file", error in (no error)=w642) -> (queue out=w639:refnum<queue>, error out=w641:errorcluster)  [unwired: 1 in, 1 out]
            n340 = Enqueue Element(queue=w639, element="connect", error in (no error)=w641) -> ()  [unwired: 1 in, 3 out]
          }
          frame "lock settings" {
            n341 = local read "device type"() -> (w653:T6)
            n342 = case shown="1002, 1502, 1902, 2002, 2502" w653 {
              tunnel: T17."Disabled and Grayed Out" ("Disabled") -> [w656 w657]
              frame 1004, 1504, 1904, 2004, 2504, Default {
                n343 = property on="settings 4ch" class="Clust (strict)"("DisabledEnum"=w656) -> ()  [unwired: 2 in, 2 out]
              }
              frame 1002, 1502, 1902, 2002, 2502 {
                n344 = property on="settings 2ch" class="Clust (strict)"("DisabledEnum"=w657) -> ()  [unwired: 2 in, 2 out]
              }
            }
            n345 = property on="butUnlockSett" class="Bool"("Visible"=TRUE) -> ()  [unwired: 2 in, 2 out]
          }
          frame "reconnect" {
            n346 = call <vilib>:"Acquire Semaphore.vi"("semaphore"=w662) -> ("error out"=w666:errorcluster, "semaphore out"=w667:T13)  [unwired: 4 in, 1 out]
            n347 = local read "abacus VISA"() -> (w663:refnum<visa-resource-name>)
            n348 = call <instrlib>:"Find Devices.vi"("error in (no error)"=w666) -> ("error out"=w659:errorcluster, "Abacus VISAs"=w665:refnum<visa-resource-name>[])  [unwired: 8 in, 1 out]
            n349 = Search 1D Array(1D array=w665, element=w663) -> (index of element=w664:i32)  [unwired: 1 in]
            n350 = Less Than 0?(x=w664) -> (x < 0?=w661:bool)
            n351 = call <vilib>:"Release Semaphore.vi"("error in (no error)"=w659, "semaphore"=w667) -> ()  [unwired: 4 in, 2 out]
            n352 = case "connection still lost?" shown="False" w661 {
              tunnel: w660 -> [w672 _]
              tunnel: [w669 _] -> w658
              frame False {
                # "when port is back"
                n353 = Flush Queue(queue=w672) -> (queue out=w671:refnum<queue>, error out=w670:errorcluster)  [unwired: 1 in, 1 out]
                n354 = Enqueue Element(queue=w671, element="reconnect step 2", error in (no error)=w670) -> (error out=w669:errorcluster)  [unwired: 1 in, 2 out]
              }
              frame True {
                # "do nothing if port not found"
              }
            }
            n355 = flat-sequence {
              tunnel: w658 -> [_]
              frame #0 {
                n356 = Get Date/Time In Seconds() -> (seconds since 1Jan1904=→"timer-reconnect":timestamp)
              }
            }
          }
          frame "reconnect step 2" {
            n357 = local read "connection state"() -> (w691:T8)
            n358 = local read "abacus VISA"() -> (w676:refnum<visa-resource-name>)
            n359 = call <vilib>:"Acquire Semaphore.vi"("semaphore"=w695) -> ("error out"=w693:errorcluster, "semaphore out"=w692:T13)  [unwired: 4 in, 1 out]
            n360 = call <instrlib>:"Open.vi"("error in (no error)"=w693, "VISA resource name"=w676) -> ("error out"=w694:errorcluster)  [unwired: 8 in, 1 out]
            n361 = call <vilib>:"Release Semaphore.vi"("error in (no error)"=w694, "semaphore"=w692) -> ("error out"=w689:errorcluster)  [unwired: 4 in, 1 out]
            n362 = case shown="\"acquisition error\"" w691 {
              selector: w691 -> [w696 w697 w698 _ w703]
              tunnel: w690 -> [_ _ _ w701 w712]
              tunnel: w689 -> [_ _ _ w700 w711]
              tunnel: [w696 w697 w698 w699 w703] -> w688
              frame "disconnected", Default {
              }
              frame "connected" {
              }
              frame "acquiring data" {
              }
              frame "connection error" {
                w699 = connectionState."connected" ("connection state")
                n363 = Enqueue Element(queue=w701, element="set settings", error in (no error)=w700) -> ()  [unwired: 1 in, 3 out]
                n364 = local write "connection state"(w699) -> ()
              }
              frame "acquisition error" {
                n365 = Enqueue Element(queue=w712, element="set settings", error in (no error)=w711) -> (queue out=w710:refnum<queue>, error out=w708:errorcluster)  [unwired: 1 in, 1 out]
                n366 = Enqueue Element(queue=w710, element="reset timers", error in (no error)=w708) -> (queue out=w709:refnum<queue>, error out=w707:errorcluster)  [unwired: 1 in, 1 out]
                n367 = Enqueue Element(queue=w709, element="start acquisition", error in (no error)=w707) -> ()  [unwired: 1 in, 3 out]
              }
            }
            n368 = local read "device type"() -> (w674:T6)
            n369 = call <instrlib>:"connectionStatusString.vi"("connected? [T]"=TRUE, "device type"=w674, "Abacus VISA"=w676) -> ("String"=w677:string)  [unwired: 8 in]
            n370 = call <vilib>:"Acquire Semaphore.vi"("semaphore"=w679) -> ("error out"=w684:errorcluster, "semaphore out"=w683:T13)  [unwired: 4 in, 1 out]
            n371 = property on="path-settings" class="Path"(error in=w684) -> (error out=w681:errorcluster, "Value"=w682:path)  [unwired: 1 in, 1 out]
            n372 = local read "delimiter"() -> (w678:string)
            n373 = local read "ref ctrls"() -> (w687:T1)
            n374 = call <instrlib>:"writeSettingsFile4ch.vi"("delimiter (,)"=w678, "message (overrides settings)"=w677, "error in (no error)"=w681, "path"=w682) -> ("error out"=w680:errorcluster)  [unwired: 6 in, 1 out]
            n375 = call <vilib>:"Release Semaphore.vi"("error in (no error)"=w680, "semaphore"=w683) -> ()  [unwired: 4 in, 2 out]
            n376 = call <instrlib>:"prependTimestamp.vi"("string in"=w677) -> ("string out"=w685:string)  [unwired: 14 in]
            n377 = call <instrlib>:"controlVisibility4Ch.vi"("device type [AB1004]"=w674, "ref controls"=w687, "connection state"=w688) -> ()  [unwired: 9 in]
            n378 = property on="status" class="Str"("Text.TextColor"=u32 0, "Value"=w685) -> ()  [unwired: 2 in, 2 out]
          }
          frame "rename files" {
            n379 = call <vilib>:"Acquire Semaphore.vi"("semaphore"=w744) -> ("error out"=w742:errorcluster, "semaphore out"=w743:T13)  [unwired: 4 in, 1 out]
            n380 = property on="path-file" class="Path"(error in=w742) -> (error out=w738:errorcluster, "Value"=w741:path)  [unwired: 1 in, 1 out]
            n381 = property on="path-fileOld" class="Path"(error in=w738, "Value"=w741) -> (error out=w713:errorcluster)  [unwired: 1 in, 1 out]
            n382 = local read "default settings"() -> (w717:T7)
            n383 = property on="path-settings" class="Path"(error in=w713) -> (error out=w715:errorcluster, "Value"=w714:path)  [unwired: 1 in, 1 out]
            n384 = property on="path-settingsOld" class="Path"(error in=w715, "Value"=w714) -> (error out=w729:errorcluster)  [unwired: 1 in, 1 out]
            n385 = Unbundle By Name(w717) -> ("settings_suffix"=w716:string)
            n386 = property on="path-new" class="Path"(error in=w729) -> (error out=w737:errorcluster, "Value"=w740:path)  [unwired: 1 in, 1 out]
            n387 = property on="path-file" class="Path"(error in=w737, "Value"=w740) -> (error out=w736:errorcluster)  [unwired: 1 in, 1 out]
            n388 = call <instrlib>:"settingsSuffixPath.vi"("settings suffix (_settings)"=w716, "path in"=w740) -> ("path out"=w739:path)  [unwired: 2 in]
            n389 = property on="path-settings" class="Path"(error in=w736, "Value"=w739) -> (error out=w725:errorcluster)  [unwired: 1 in, 1 out]
            n390 = property on="path-fileOld" class="Path"(error in=w725) -> ("Value"=w733:path)  [unwired: 1 in, 2 out]
            n391 = property on="path-file" class="Path"(error in=w725) -> (error out=w723:errorcluster, "Value"=w724:path)  [unwired: 1 in, 1 out]
            n392 = call <vilib>:"Is Path and Not Empty.vi"("path"=w733) -> ("Is Path and Not Empty?"=w731:bool)  [unwired: 4 in]
            n393 = call <vilib>:"Check if File or Folder Exists.vi"("error in (no error)"=w723, "path"=w733) -> ("error out"=w728:errorcluster, "file or folder exists?"=w732:bool)  [unwired: 7 in, 1 out]
            n394 = And(x=w731, y=w732) -> (x .and. y?=w735:bool)
            n395 = case "rename file if exists" shown="True" w735 {
              tunnel: w733 -> [_ w754]
              tunnel: w724 -> [_ w753]
              tunnel: w728 -> [w750 w752]
              tunnel: [w750 w751] -> w722
              frame False {
              }
              frame True {
                n396 = Move(source path=w754, error in=w752, 10:w753) -> (error out=w751:errorcluster)  [unwired: 2 in, 2 out]
              }
            }
            n397 = property on="path-settingsOld" class="Path"(error in=w722) -> ("Value"=w730:path)  [unwired: 1 in, 2 out]
            n398 = property on="path-settings" class="Path"(error in=w722) -> (error out=w720:errorcluster, "Value"=w721:path)  [unwired: 1 in, 1 out]
            n399 = call <vilib>:"Check if File or Folder Exists.vi"("error in (no error)"=w720, "path"=w730) -> ("error out"=w727:errorcluster, "file or folder exists?"=w718:bool)  [unwired: 7 in, 1 out]
            n400 = call <vilib>:"Is Path and Not Empty.vi"("path"=w730) -> ("Is Path and Not Empty?"=w719:bool)  [unwired: 4 in]
            n401 = And(x=w719, y=w718) -> (x .and. y?=w734:bool)
            n402 = case "rename file if exists" shown="True" w734 {
              tunnel: w721 -> [_ w749]
              tunnel: w730 -> [_ w748]
              tunnel: w727 -> [w745 w747]
              tunnel: [w745 w746] -> w726
              frame False {
              }
              frame True {
                n403 = Move(source path=w748, error in=w747, 10:w749) -> (error out=w746:errorcluster)  [unwired: 2 in, 2 out]
              }
            }
            n404 = call <vilib>:"Release Semaphore.vi"("error in (no error)"=w726, "semaphore"=w743) -> ()  [unwired: 4 in, 2 out]
          }
          frame "reset controls" {
            w766 = connectionState."disconnected" ("connection state")
            n405 = control-ref of="butConnect"() -> (w761:refnum<vi>)
            n406 = control-ref of="butDisconnect"() -> (w762:refnum<vi>)
            n407 = control-ref of="butStartAcq"() -> (w763:refnum<vi>)
            n408 = control-ref of="butStopAcq"() -> (w764:refnum<vi>)
            n409 = control-ref of="butLoadDefSett"() -> (w760:refnum<vi>)
            n410 = control-ref of="butUnlockSett"() -> (w759:refnum<vi>)
            n411 = control-ref of="settings 2ch"() -> (w755:refnum<vi>)
            n412 = control-ref of="settings 4ch"() -> (w756:refnum<vi>)
            n413 = Bundle(cluster=T1 {"butConnect"=refnum, "butDisconnect"=refnum, "butStartAcq"=refnum, "butStopAcq"=refnum, "butLoadDefSett"=refnum, "butUnlockSett"=refnum, "settings 2ch"=refnum, "settings 4ch"=refnum} ("ref ctrls 2"), "butConnect"=w761, "butDisconnect"=w762, "butStartAcq"=w763, "butStopAcq"=w764, "butLoadDefSett"=w760, "butUnlockSett"=w759, "settings 2ch"=w755, "settings 4ch"=w756) -> (w757:T1)
            "ref ctrls" <- w757
            n414 = local read "device type"() -> (w765:T6)
            n415 = call <instrlib>:"controlVisibility4Ch.vi"("device type [AB1004]"=w765, "ref controls"=w757, "connection state"=w766) -> ()  [unwired: 9 in]
            "connection state" <- w766
          }
          frame "reset indicators" {
            n416 = control-ref of="graph-A"() -> (w773:refnum<vi>)
            n417 = control-ref of="graph-B"() -> (w775:refnum<vi>)
            n418 = control-ref of="graph-C"() -> (w777:refnum<vi>)
            n419 = control-ref of="graph-D"() -> (w779:refnum<vi>)
            n420 = control-ref of="dataTable"() -> (w771:refnum<vi>)
            n421 = control-ref of="counters 2ch"() -> (w767:refnum<vi>)
            n422 = control-ref of="graph coinc"() -> (w772:refnum<vi>)
            n423 = control-ref of="graph-A-S"() -> (w774:refnum<vi>)
            n424 = control-ref of="graph-B-S"() -> (w776:refnum<vi>)
            n425 = control-ref of="graph-C-S"() -> (w778:refnum<vi>)
            n426 = control-ref of="graph-D-S"() -> (w780:refnum<vi>)
            n427 = control-ref of="counters 4ch"() -> (w770:refnum<vi>)
            n428 = Bundle("counters 2ch"=w767, "counters 4ch"=w770, "dataTable"=w771, "graph coinc"=w772, "graph-A"=w773, "graph-A-S"=w774, "graph-B"=w775, "graph-B-S"=w776, "graph-C"=w777, "graph-C-S"=w778, "graph-D"=w779, "graph-D-S"=w780) -> (w769:T2)  [unwired: 1 in]
            "ref indics" <- w769
            n429 = local read "device type"() -> (w768:T6)
            n430 = call <instrlib>:"indicatorVisibility4Ch.vi"("device type [AB1004]"=w768, "ref indics"=w769) -> ()  [unwired: 10 in]
          }
          frame "reset timers" {
            n431 = local read "dataTable"() -> (w782:string[][])
            n432 = local read "settings 4ch"() -> (w789:T4)
            n433 = Empty Array?(array=w782) -> (empty?=w781:bool)
            n434 = Get Date/Time In Seconds() -> (seconds since 1Jan1904=w785:timestamp)
            n435 = case shown="True" w781 {
              tunnel: w785 -> [_ w790]
              frame False {
              }
              frame True {
                "timer-begin" <- w790
              }
            }
            n436 = Unbundle By Name(w789) -> ("sampling"=w787:u32)
            n437 = local write "timer-current"(w785) -> ()
            n438 = local write "timer-lastRead"(w785) -> ()
            n439 = To Double Precision Float(number=w787) -> (double precision float=w786:dbl)
            n440 = Divide(x=w786, y=1000.0) -> (x/y=w784:dbl)
            n441 = Add(x=w785, y=w784) -> (x+y=w783:timestamp)
            n442 = local write "timer-nextRead"(w783) -> ()
          }
          frame "reset values" {
            n443 = stacked-sequence {
              frame #0 {
                w793 = T6 1004 items=["any"=0, "AB1002"=1002, "AB1004"=1004] ("device type")
                # "Clear any data indicators"
                n444 = property on="dataTable" class="Tbl (strict)"("Value"=string[][] [] ("dataTable"), "Index Values"=T19 {"Row"=0, "Column"=0}) -> ()  [unwired: 2 in, 2 out]
                n445 = local write "device type"(w793) -> ()
                n446 = property on="counters 2ch" class="Clust (strict)"("Value"=T10 {"counter_A"=0, "counter_B"=0, "counter_AB"=0, "counters_ID"=0, "time_left"=0} ("counters 2ch")) -> ()  [unwired: 2 in, 2 out]
                n447 = call <instrlib>:"prependTimestamp.vi"("string in"="Session started. Please connect to a device.") -> ("string out"=w796:string)  [unwired: 14 in]
                n448 = local write "error"(errorcluster {"status"=FALSE, "code"=0, "source"=""} ("error constant")) -> ()
                n449 = property on="status" class="Str"("Text.TextColor"=u32 0, "Value"=w796) -> ()  [unwired: 2 in, 2 out]
                n450 = property on="counters 4ch" class="Clust (strict)"("Value"=T18 {"counter_A"=0, "counter_B"=0, "counter_C"=0, "counter_D"=0, "counter_AB"=0, "counter_AC"=0, "counter_AD"=0, "counter_BC"=0, "counter_BD"=0, "counter_CD"=0, "counter_multiple_1"=0, "counters_ID"=0, "time_left"=0}) -> ()  [unwired: 2 in, 2 out]
              }
              frame #1 {
                w801 = cluster{timestamp[], u32[]} {[], []} ("graph-A-S")
                n451 = property on="graph-A-S" class="XYGraph (strict)"("Value"=w801) -> ()  [unwired: 2 in, 2 out]
                n452 = property on="graph-A" class="XYGraph (strict)"("Value"=w801) -> ()  [unwired: 2 in, 2 out]
                n453 = property on="graph-B-S" class="XYGraph (strict)"("Value"=w801) -> ()  [unwired: 2 in, 2 out]
                n454 = property on="graph-B" class="XYGraph (strict)"("Value"=w801) -> ()  [unwired: 2 in, 2 out]
                n455 = property on="graph-C" class="XYGraph (strict)"("Value"=w801) -> ()  [unwired: 2 in, 2 out]
                n456 = property on="graph-C-S" class="XYGraph (strict)"("Value"=w801) -> ()  [unwired: 2 in, 2 out]
                n457 = property on="graph-D" class="XYGraph (strict)"("Value"=w801) -> ()  [unwired: 2 in, 2 out]
                n458 = property on="graph-D-S" class="XYGraph (strict)"("Value"=w801) -> ()  [unwired: 2 in, 2 out]
                n459 = property on="graph coinc" class="XYGraph (strict)"("Value"=cluster{timestamp[], u32[]}[] [] ("graph coinc")) -> ()  [unwired: 2 in, 2 out]
              }
              frame #2 {
                # "'default settings' cluster is set"
                n460 = Current VI's Path() -> (path=w806:path)
                n461 = Strip Path(path=w806) -> (stripped path=w807:path)  [unwired: 1 out]
                n462 = Build Path(base path=w807, name or relative path="settings.py" ("Path")) -> (appended path=w808:path)
                "path-defsettings" <- w808
                n463 = call <vilib>:"Check if File or Folder Exists.vi"("path"=w808) -> ("file or folder exists?"=w804:bool, "dup path"=w805:path)  [unwired: 8 in, 1 out]
                n464 = case shown="True" w804 {
                  tunnel: w805 -> [w810 w812]
                  tunnel: [w809 w811] -> w802
                  frame False {
                    n465 = call <instrlib>:"writeSettingsPy.vi"("Path"=w810) -> ("default settings out"=w809:T7)  [unwired: 9 in, 1 out]
                  }
                  frame True {
                    n466 = call <instrlib>:"readSettingsPy.vi"("Path"=w812) -> ("default settings"=w811:T7)  [unwired: 10 in]
                  }
                }
                n467 = property on="default settings" class="Clust (strict)"("Value"=w802) -> ()  [unwired: 2 in, 2 out]
              }
              frame #3 {
                # "Path construction"
                n468 = local read "default settings"() -> (w815:T7)
                n469 = call <instrlib>:"buildDefaultPath.vi"("default settings"=w815) -> ("settings path"=w813:path, "data path"=w814:path)  [unwired: 3 in]
                n470 = local write "path-file"(w814) -> ()
                n471 = local write "path-settings"(w813) -> ()
              }
              frame #4 {
                n472 = local read "default settings"() -> (w818:T7)
                n473 = Unbundle By Name(w818) -> ("delimiter"=w816:string)
                n474 = case shown="\",\", \";\", Default" w816 {
                  selector: w816 -> [_ _ w821]
                  tunnel: [w819 "\t" w821] -> w817
                  frame "Space", "space" {
                    n475 = call <vilib>:"Space Constant.vi"() -> ("String"=w819:string)
                  }
                  frame "Tab", "tab" {
                  }
                  frame ",", ";", Default {
                  }
                }
                "delimiter" <- w817
              }
              frame #5 {
                n476 = local read "default settings"() -> (w823:T7)
                n477 = Unbundle By Name(w823) -> ("Abacus settings"=w822:T4)
                n478 = call <instrlib>:"Settings4ch To Settings2ch.vi"("settings4ch"=w822) -> ("settings2ch"=w824:T3)
                n479 = local write "settings 2ch"(w824) -> ()
                n480 = local write "settings 4ch"(w822) -> ()
                n481 = local write "settings_old"(w822) -> ()
              }
            }
          }
          frame "set coincidence window" {
            n482 = property on="settings_old" class="Clust (strict)"() -> (error out=w835:errorcluster, "Value"=w842:T21)  [unwired: 2 in, 1 out]
            n483 = call <vilib>:"Acquire Semaphore.vi"("error in (no error)"=w835, "semaphore"=w843) -> ("error out"=w849:errorcluster, "semaphore out"=w850:T13)  [unwired: 3 in, 1 out]
            n484 = local read "abacus VISA"() -> (w848:refnum<visa-resource-name>)
            n485 = local read "device type"() -> (w830:T6)
            n486 = property on="coincidence_window" class="DigNum (strict)"(error in=w849) -> (error out=w847:errorcluster, "Value"=w826:u32)  [unwired: 1 in, 1 out]
            n487 = Format Into String(initial string="Coincidence window set to " ("string in"), w826, "ns." ("string in")) -> (resulting string=w825:string)  [unwired: 2 in, 1 out]
            n488 = call <instrlib>:"Configure Coincidence Window.vi"("device type"=w830, "error in (no error)"=w847, "value ns (10ns)"=w826, "VISA Refnum in"=w848) -> ("error out"=w845:errorcluster, "value ns out"=w846:u32)  [unwired: 5 in, 1 out]
            n489 = call <instrlib>:"prependTimestamp.vi"("string in"=w825) -> ("string out"=w829:string)  [unwired: 14 in]
            n490 = property on="coincidence_window" class="DigNum (strict)"(error in=w845, "Value"=w846) -> (error out=w844:errorcluster)  [unwired: 1 in, 1 out]
            n491 = local write "status"(w829) -> ()
            n492 = call <vilib>:"Release Semaphore.vi"("error in (no error)"=w844, "semaphore"=w850) -> ("error out"=w833:errorcluster)  [unwired: 4 in, 1 out]
            n493 = call <vilib>:"Acquire Semaphore.vi"("semaphore"=w834) -> ("error out"=w841:errorcluster, "semaphore out"=w840:T13)  [unwired: 4 in, 1 out]
            n494 = property on="settings 4ch" class="Clust (strict)"(error in=w833) -> (error out=w832:errorcluster, "Value"=w831:T21)  [unwired: 1 in, 1 out]
            n495 = case shown="No Error" w833 {
              frame No Error {
                n496 = Get Date/Time In Seconds() -> (seconds since 1Jan1904=w851:timestamp)
                n497 = local write "timer-settings"(w851) -> ()
              }
              frame Error {
              }
            }
            n498 = property on="path-settings" class="Path"(error in=w841) -> (error out=w838:errorcluster, "Value"=w837:path)  [unwired: 1 in, 1 out]
            n499 = local read "delimiter"() -> (w836:string)
            n500 = call <instrlib>:"writeSettingsFile4ch.vi"("delimiter (,)"=w836, "error in (no error)"=w838, "old settings"=w842, "new settings"=w831, "path"=w837) -> ("error out"=w839:errorcluster)  [unwired: 5 in, 1 out]
            n501 = property on="settings_old" class="Clust (strict)"(error in=w832, "Value"=w831) -> ()  [unwired: 1 in, 2 out]
            n502 = call <vilib>:"Release Semaphore.vi"("error in (no error)"=w839, "semaphore"=w840) -> ()  [unwired: 4 in, 2 out]
          }
          frame "set default settings" {
            n503 = local read "connection state"() -> (w855:T8)
            n504 = case shown="\"connected\", \"acquiring data\"" w855 {
              tunnel: w854 -> [_ w868]
              tunnel: w853 -> [_ w869]
              tunnel: w852 -> [_ w856]
              frame "disconnected", Default {
              }
              frame "connected", "acquiring data" {
                n505 = local read "default settings"() -> (w875:T7)
                n506 = local read "device type"() -> (w871:T6)
                n507 = Unbundle By Name(w875) -> ("Abacus settings"=w876:T4)
                n508 = property on="settings_old" class="Clust (strict)"(error in=w868) -> (error out=w867:errorcluster, "Value"=w857:T21)  [unwired: 1 in, 1 out]
                n509 = case shown="1002, 1502, 1902, 2002, 2502" w871 {
                  tunnel: w876 -> [w884 w888]
                  tunnel: [w883 w886] -> w877
                  tunnel: [w882 w885] -> w878
                  frame 1004, 1504, 1904, Default {
                    n510 = call <instrlib>:"Unbundle by Name Settings 4ch.vi"("input cluster settings 4ch"=w884) -> ("names"=w882:string[], "values"=w883:u32[])  [unwired: 13 in]
                  }
                  frame 1002, 1502, 1902, 2002, 2502 {
                    n511 = call <instrlib>:"Settings4ch To Settings2ch.vi"("settings4ch"=w888) -> ("settings2ch"=w887:T3)
                    n512 = call <instrlib>:"Unbundle by Name Settings 2ch.vi"("input cluster settings 2ch"=w887) -> ("names"=w885:string[], "values"=w886:u32[])  [unwired: 13 in]
                  }
                }
                n513 = local read "abacus VISA"() -> (w870:refnum<visa-resource-name>)
                n514 = call <instrlib>:"prependTimestamp.vi"("string in"="Default settings loaded.") -> ("string out"=w879:string)  [unwired: 14 in]
                n515 = local write "status"(w879) -> ()
                n516 = call <vilib>:"Acquire Semaphore.vi"("error in (no error)"=w867, "semaphore"=w869) -> ("error out"=w874:errorcluster, "semaphore out"=w873:T13)  [unwired: 3 in, 1 out]
                n517 = call <instrlib>:"Configure By Name.vi"("device type"=w871, "error in (no error)"=w874, "values"=w877, "labels"=w878, "VISA Refnum in"=w870) -> ("error out"=w872:errorcluster)  [unwired: 5 in, 1 out]
                n518 = local read "delimiter"() -> (w861:string)
                n519 = call <vilib>:"Release Semaphore.vi"("error in (no error)"=w872, "semaphore"=w873) -> ("error out"=w858:errorcluster)  [unwired: 4 in, 1 out]
                n520 = call <vilib>:"Acquire Semaphore.vi"("error in (no error)"=w858, "semaphore"=w856) -> ("error out"=w866:errorcluster, "semaphore out"=w865:T13)  [unwired: 3 in, 1 out]
                n521 = case shown="No Error" w858 {
                  frame No Error {
                    n522 = Get Date/Time In Seconds() -> (seconds since 1Jan1904=w881:timestamp)
                    n523 = local write "timer-settings"(w881) -> ()
                  }
                  frame Error {
                  }
                }
                n524 = property on="path-settings" class="Path"(error in=w866) -> (error out=w863:errorcluster, "Value"=w862:path)  [unwired: 1 in, 1 out]
                n525 = property on="settings 4ch" class="Clust (strict)"(error in=w858) -> (error out=w860:errorcluster, "Value"=w859:T21)  [unwired: 1 in, 1 out]
                n526 = call <instrlib>:"writeSettingsFile4ch.vi"("delimiter (,)"=w861, "error in (no error)"=w863, "old settings"=w857, "new settings"=w859, "path"=w862) -> ("error out"=w864:errorcluster)  [unwired: 5 in, 1 out]
                n527 = property on="settings_old" class="Clust (strict)"(error in=w860, "Value"=w859) -> ()  [unwired: 1 in, 2 out]
                n528 = call <vilib>:"Release Semaphore.vi"("error in (no error)"=w864, "semaphore"=w865) -> ()  [unwired: 4 in, 2 out]
              }
            }
          }
          frame "set delay A".."set delay Z" {
            w911 = T23 0 items=["none", "A", "B", "C", "D", "E", "F", "G", "H"] ("channel")
            n529 = property on="settings_old" class="Clust (strict)"() -> (error out=w899:errorcluster, "Value"=w906:T21)  [unwired: 2 in, 1 out]
            n530 = call <instrlib>:"getLastChar.vi"("string"=w908) -> ("last char"=w889:string)
            n531 = call <instrlib>:"letterToNumber.vi"("letter"=w889) -> ("number"=w910:u8)
            n532 = call <vilib>:"Acquire Semaphore.vi"("error in (no error)"=w899, "semaphore"=w907) -> ("error out"=w917:errorcluster, "semaphore out"=w918:T13)  [unwired: 3 in, 1 out]
            n533 = Type Cast(type=w911, x=w910) -> (*(type *) &x=w909:T23)
            n534 = local read "abacus VISA"() -> (w916:refnum<visa-resource-name>)
            n535 = local read "device type"() -> (w919:T6)
            n536 = case shown="1" w909 {
              tunnel: w917 -> [w934 w937 w940 w943 w946]
              tunnel: [_ w936 w939 w942 w945] -> w915
              tunnel: [w934 w935 w938 w941 w944] -> w914
              frame 0, Default {
              }
              frame 1 {
                n537 = property on="delay_A" class="DigNum (strict)"(error in=w937) -> (error out=w935:errorcluster, "Value"=w936:u32)  [unwired: 1 in, 1 out]
              }
              frame 2 {
                n538 = property on="delay_B" class="DigNum (strict)"(error in=w940) -> (error out=w938:errorcluster, "Value"=w939:u32)  [unwired: 1 in, 1 out]
              }
              frame 3 {
                n539 = property on="delay_C" class="DigNum (strict)"(error in=w943) -> (error out=w941:errorcluster, "Value"=w942:u32)  [unwired: 1 in, 1 out]
              }
              frame 4 {
                n540 = property on="delay_D" class="DigNum (strict)"(error in=w946) -> (error out=w944:errorcluster, "Value"=w945:u32)  [unwired: 1 in, 1 out]
              }
            }
            n541 = call <instrlib>:"Configure Delay.vi"("device type"=w919, "error in (no error)"=w914, "value (0 ns)"=w915, "channel"=w909, "VISA Refnum in"=w916) -> ("error out"=w913:errorcluster, "value ns out"=w891:u32)  [unwired: 4 in, 1 out]
            n542 = Format Into String(initial string="Delay set to " ("string in"), w891, "ns in channel" ("string in"), w889) -> (resulting string=w894:string)  [unwired: 2 in, 1 out]
            n543 = call <instrlib>:"prependTimestamp.vi"("string in"=w894) -> ("string out"=w893:string)  [unwired: 14 in]
            n544 = case shown="1" w909 {
              tunnel: w891 -> [_ w924 w927 w930 w933]
              tunnel: w913 -> [w921 w923 w926 w929 w932]
              tunnel: [w921 w922 w925 w928 w931] -> w912
              frame 0, Default {
              }
              frame 1 {
                n545 = property on="delay_A" class="DigNum (strict)"(error in=w923, "Value"=w924) -> (error out=w922:errorcluster)  [unwired: 1 in, 1 out]
              }
              frame 2 {
                n546 = property on="delay_B" class="DigNum (strict)"(error in=w926, "Value"=w927) -> (error out=w925:errorcluster)  [unwired: 1 in, 1 out]
              }
              frame 3 {
                n547 = property on="delay_C" class="DigNum (strict)"(error in=w929, "Value"=w930) -> (error out=w928:errorcluster)  [unwired: 1 in, 1 out]
              }
              frame 4 {
                n548 = property on="delay_D" class="DigNum (strict)"(error in=w932, "Value"=w933) -> (error out=w931:errorcluster)  [unwired: 1 in, 1 out]
              }
            }
            n549 = local write "status"(w893) -> ()
            n550 = call <vilib>:"Acquire Semaphore.vi"("semaphore"=w898) -> ("error out"=w905:errorcluster, "semaphore out"=w904:T13)  [unwired: 4 in, 1 out]
            n551 = call <vilib>:"Release Semaphore.vi"("error in (no error)"=w912, "semaphore"=w918) -> ("error out"=w895:errorcluster)  [unwired: 4 in, 1 out]
            n552 = case shown="No Error" w895 {
              frame No Error {
                n553 = Get Date/Time In Seconds() -> (seconds since 1Jan1904=w920:timestamp)
                n554 = local write "timer-settings"(w920) -> ()
              }
              frame Error {
              }
            }
            n555 = property on="path-settings" class="Path"(error in=w905) -> (error out=w902:errorcluster, "Value"=w901:path)  [unwired: 1 in, 1 out]
            n556 = local read "delimiter"() -> (w900:string)
            n557 = property on="settings 4ch" class="Clust (strict)"(error in=w895) -> (error out=w897:errorcluster, "Value"=w896:T21)  [unwired: 1 in, 1 out]
            n558 = call <instrlib>:"writeSettingsFile4ch.vi"("delimiter (,)"=w900, "error in (no error)"=w902, "old settings"=w906, "new settings"=w896, "path"=w901) -> ("error out"=w903:errorcluster)  [unwired: 5 in, 1 out]
            n559 = property on="settings_old" class="Clust (strict)"(error in=w897, "Value"=w896) -> ()  [unwired: 1 in, 2 out]
            n560 = call <vilib>:"Release Semaphore.vi"("error in (no error)"=w903, "semaphore"=w904) -> ()  [unwired: 4 in, 2 out]
          }
          frame "set multi 1".."set multi 9" {
            w966 = u8 0  # U8
            n561 = property on="settings_old" class="Clust (strict)"() -> (error out=w955:errorcluster, "Value"=w962:T21)  [unwired: 2 in, 1 out]
            n562 = property on="config_multiple_1" class="Ring (strict)"() -> ("RingText.Text"=w949:string)  [unwired: 2 in, 2 out]
            n563 = call <instrlib>:"getLastChar.vi"("string"=w963) -> ("last char"=w967:string)
            n564 = Decimal String To Number(string=w967, default (0L)=w966) -> (number=w972:u8)  [unwired: 1 in, 1 out]
            n565 = call <vilib>:"Acquire Semaphore.vi"("error in (no error)"=w955, "semaphore"=w964) -> ("error out"=w969:errorcluster, "semaphore out"=w968:T13)  [unwired: 3 in, 1 out]
            n566 = case shown="1" w972 {
              tunnel: w969 -> [w981 w984]
              tunnel: [w981 w983] -> w970
              tunnel: [_ w982] -> w971
              frame 0, Default {
              }
              frame 1 {
                n567 = property on="config_multiple_1" class="Ring (strict)"(error in=w984) -> (error out=w983:errorcluster, "Value"=w982:T22)  [unwired: 1 in, 1 out]
              }
            }
            n568 = Concatenate Strings("Multi-fold set to " ("string in"), w949) -> (w950:string)
            n569 = case shown="1..8" w972 {
              selector: w972 -> [_ w975]
              tunnel: [w974 w980] -> w965
              tunnel: w970 -> [w974 w977]
              tunnel: w971 -> [_ w976]
              frame 0, Default {
              }
              frame 1..8 {
                n570 = local read "abacus VISA"() -> (w978:refnum<visa-resource-name>)
                n571 = local read "device type"() -> (w979:T6)
                n572 = call <instrlib>:"Configure Multiple Coincidence.vi"("device type"=w979, "error in (no error)"=w977, "Multiple coincidence configuration"=w976, "multi-fold counter (1)"=w975, "VISA Refnum in"=w978) -> ("error out"=w980:errorcluster)  [unwired: 5 in, 1 out]
              }
            }
            n573 = call <instrlib>:"prependTimestamp.vi"("string in"=w950) -> ("string out"=w947:string)  [unwired: 14 in]
            n574 = local write "status"(w947) -> ()
            n575 = call <vilib>:"Acquire Semaphore.vi"("semaphore"=w954) -> ("error out"=w961:errorcluster, "semaphore out"=w960:T13)  [unwired: 4 in, 1 out]
            n576 = call <vilib>:"Release Semaphore.vi"("error in (no error)"=w965, "semaphore"=w968) -> ("error out"=w952:errorcluster)  [unwired: 4 in, 1 out]
            n577 = case shown="No Error" w952 {
              frame No Error {
                n578 = Get Date/Time In Seconds() -> (seconds since 1Jan1904=w973:timestamp)
                n579 = local write "timer-settings"(w973) -> ()
              }
              frame Error {
              }
            }
            n580 = property on="path-settings" class="Path"(error in=w961) -> (error out=w958:errorcluster, "Value"=w957:path)  [unwired: 1 in, 1 out]
            n581 = local read "delimiter"() -> (w956:string)
            n582 = property on="settings 4ch" class="Clust (strict)"(error in=w952) -> (error out=w953:errorcluster, "Value"=w951:T21)  [unwired: 1 in, 1 out]
            n583 = call <instrlib>:"writeSettingsFile4ch.vi"("delimiter (,)"=w956, "error in (no error)"=w958, "old settings"=w962, "new settings"=w951, "path"=w957) -> ("error out"=w959:errorcluster)  [unwired: 5 in, 1 out]
            n584 = property on="settings_old" class="Clust (strict)"(error in=w953, "Value"=w951) -> ()  [unwired: 1 in, 2 out]
            n585 = call <vilib>:"Release Semaphore.vi"("error in (no error)"=w959, "semaphore"=w960) -> ()  [unwired: 4 in, 2 out]
          }
          frame "set sampling" {
            n586 = property on="settings_old" class="Clust (strict)"() -> (error out=w997:errorcluster, "Value"=w994:T21)  [unwired: 2 in, 1 out]
            n587 = call <vilib>:"Acquire Semaphore.vi"("error in (no error)"=w997, "semaphore"=w1004) -> ("error out"=w1009:errorcluster, "semaphore out"=w1010:T13)  [unwired: 3 in, 1 out]
            n588 = local read "abacus VISA"() -> (w1008:refnum<visa-resource-name>)
            n589 = local read "device type"() -> (w990:T6)
            n590 = property on="sampling" class="Ring (strict)"(error in=w1009) -> (error out=w1006:errorcluster, "Value"=w1007:u32)  [unwired: 1 in, 1 out]
            n591 = call <instrlib>:"Configure Sampling Time.vi"("device type"=w990, "error in (no error)"=w1006, "value (1000 ms)"=w1007, "VISA Refnum in"=w1008) -> ("error out"=w1005:errorcluster, "value ms out"=w985:u32)  [unwired: 5 in, 1 out]
            n592 = Format Into String(initial string="Sampling set to " ("string in"), w985, "ms." ("string in")) -> (resulting string=w989:string)  [unwired: 2 in, 1 out]
            n593 = call <instrlib>:"prependTimestamp.vi"("string in"=w989) -> ("string out"=w988:string)  [unwired: 14 in]
            n594 = property on="sampling" class="Ring (strict)"(error in=w1005, "Value"=w985) -> (error out=w995:errorcluster)  [unwired: 1 in, 1 out]
            n595 = local write "status"(w988) -> ()
            n596 = call <vilib>:"Release Semaphore.vi"("error in (no error)"=w995, "semaphore"=w1010) -> ("error out"=w993:errorcluster)  [unwired: 4 in, 1 out]
            n597 = call <vilib>:"Acquire Semaphore.vi"("semaphore"=w996) -> ("error out"=w1003:errorcluster, "semaphore out"=w1002:T13)  [unwired: 4 in, 1 out]
            n598 = property on="settings 4ch" class="Clust (strict)"(error in=w993) -> (error out=w992:errorcluster, "Value"=w991:T21)  [unwired: 1 in, 1 out]
            n599 = property on="path-settings" class="Path"(error in=w1003) -> (error out=w1000:errorcluster, "Value"=w999:path)  [unwired: 1 in, 1 out]
            n600 = local read "delimiter"() -> (w998:string)
            n601 = case shown="No Error" w993 {
              frame No Error {
                n602 = Get Date/Time In Seconds() -> (seconds since 1Jan1904=w1011:timestamp)
                n603 = local write "timer-settings"(w1011) -> ()
              }
              frame Error {
              }
            }
            n604 = call <instrlib>:"writeSettingsFile4ch.vi"("delimiter (,)"=w998, "error in (no error)"=w1000, "old settings"=w994, "new settings"=w991, "path"=w999) -> ("error out"=w1001:errorcluster)  [unwired: 5 in, 1 out]
            n605 = property on="settings_old" class="Clust (strict)"(error in=w992, "Value"=w991) -> ()  [unwired: 1 in, 2 out]
            n606 = call <vilib>:"Release Semaphore.vi"("error in (no error)"=w1001, "semaphore"=w1002) -> ()  [unwired: 4 in, 2 out]
          }
          frame "set settings" {
            n607 = local read "device type"() -> (w1014:T6)
            n608 = case shown="1002, 1502, 1902, 2002, 2502" w1014 {
              tunnel: [string[] ["set sampling", "set coincidence window", "set delay A", "set delay B", "set delay C", "set delay D", "set sleep A", "set sleep B", "set sleep C", "set sleep D", "set multi 1"] string[] ["set sampling", "set coincidence window", "set delay A", "set delay B", "set sleep A", "set sleep B"]] -> w1015
              frame 1004, 1504, 1904, Default {
              }
              frame 1002, 1502, 1902, 2002, 2502 {
              }
            }
            n609 = for {
              tunnel: w1015 -> [w1018] mode=indexing
              shift-right: [w1021] -> _
              shift-left: w1012 -> [w1022]
              shift-right: [w1019] -> _
              shift-left: w1013 -> [w1020]
              n610 = Enqueue Element(queue=w1020, element=w1018, error in (no error)=w1022) -> (queue out=w1019:refnum<queue>, error out=w1021:errorcluster)  [unwired: 1 in, 1 out]
            }
          }
          frame "set sleep A".."set sleep Z" {
            w1045 = T23 0 items=["none", "A", "B", "C", "D", "E", "F", "G", "H"] ("channel")
            n611 = call <instrlib>:"getLastChar.vi"("string"=w1042) -> ("last char"=w1023:string)
            n612 = property on="settings_old" class="Clust (strict)"() -> (error out=w1033:errorcluster, "Value"=w1040:T21)  [unwired: 2 in, 1 out]
            n613 = call <instrlib>:"letterToNumber.vi"("letter"=w1023) -> ("number"=w1044:u8)
            n614 = Type Cast(type=w1045, x=w1044) -> (*(type *) &x=w1043:T23)
            n615 = call <vilib>:"Acquire Semaphore.vi"("error in (no error)"=w1033, "semaphore"=w1041) -> ("error out"=w1051:errorcluster, "semaphore out"=w1052:T13)  [unwired: 3 in, 1 out]
            n616 = local read "abacus VISA"() -> (w1050:refnum<visa-resource-name>)
            n617 = local read "device type"() -> (w1053:T6)
            n618 = case shown="1" w1043 {
              tunnel: w1051 -> [w1068 w1071 w1074 w1077 w1080]
              tunnel: [_ w1070 w1073 w1076 w1079] -> w1049
              tunnel: [w1068 w1069 w1072 w1075 w1078] -> w1048
              frame 0, Default {
              }
              frame 1 {
                n619 = property on="sleep_A" class="DigNum (strict)"(error in=w1071) -> (error out=w1069:errorcluster, "Value"=w1070:u32)  [unwired: 1 in, 1 out]
              }
              frame 2 {
                n620 = property on="sleep_B" class="DigNum (strict)"(error in=w1074) -> (error out=w1072:errorcluster, "Value"=w1073:u32)  [unwired: 1 in, 1 out]
              }
              frame 3 {
                n621 = property on="sleep_C" class="DigNum (strict)"(error in=w1077) -> (error out=w1075:errorcluster, "Value"=w1076:u32)  [unwired: 1 in, 1 out]
              }
              frame 4 {
                n622 = property on="sleep_D" class="DigNum (strict)"(error in=w1080) -> (error out=w1078:errorcluster, "Value"=w1079:u32)  [unwired: 1 in, 1 out]
              }
            }
            n623 = call <instrlib>:"Configure Sleep.vi"("device type"=w1053, "error in (no error)"=w1048, "value (0 ns)"=w1049, "channel"=w1043, "VISA Refnum in"=w1050) -> ("error out"=w1047:errorcluster, "value ns out"=w1024:u32)  [unwired: 4 in, 1 out]
            n624 = Format Into String(initial string="Sleep time set to " ("string in"), w1024, "ns in channel" ("string in"), w1023) -> (resulting string=w1028:string)  [unwired: 2 in, 1 out]
            n625 = call <instrlib>:"prependTimestamp.vi"("string in"=w1028) -> ("string out"=w1027:string)  [unwired: 14 in]
            n626 = local write "status"(w1027) -> ()
            n627 = case shown="1" w1043 {
              tunnel: w1024 -> [_ w1058 w1061 w1064 w1067]
              tunnel: w1047 -> [w1055 w1057 w1060 w1063 w1066]
              tunnel: [w1055 w1056 w1059 w1062 w1065] -> w1046
              frame 0, Default {
              }
              frame 1 {
                n628 = property on="sleep_A" class="DigNum (strict)"(error in=w1057, "Value"=w1058) -> (error out=w1056:errorcluster)  [unwired: 1 in, 1 out]
              }
              frame 2 {
                n629 = property on="sleep_B" class="DigNum (strict)"(error in=w1060, "Value"=w1061) -> (error out=w1059:errorcluster)  [unwired: 1 in, 1 out]
              }
              frame 3 {
                n630 = property on="sleep_C" class="DigNum (strict)"(error in=w1063, "Value"=w1064) -> (error out=w1062:errorcluster)  [unwired: 1 in, 1 out]
              }
              frame 4 {
                n631 = property on="sleep_D" class="DigNum (strict)"(error in=w1066, "Value"=w1067) -> (error out=w1065:errorcluster)  [unwired: 1 in, 1 out]
              }
            }
            n632 = call <vilib>:"Acquire Semaphore.vi"("semaphore"=w1032) -> ("error out"=w1039:errorcluster, "semaphore out"=w1038:T13)  [unwired: 4 in, 1 out]
            n633 = call <vilib>:"Release Semaphore.vi"("error in (no error)"=w1046, "semaphore"=w1052) -> ("error out"=w1031:errorcluster)  [unwired: 4 in, 1 out]
            n634 = case shown="No Error" w1031 {
              frame No Error {
                n635 = Get Date/Time In Seconds() -> (seconds since 1Jan1904=w1054:timestamp)
                n636 = local write "timer-settings"(w1054) -> ()
              }
              frame Error {
              }
            }
            n637 = property on="path-settings" class="Path"(error in=w1039) -> (error out=w1036:errorcluster, "Value"=w1035:path)  [unwired: 1 in, 1 out]
            n638 = local read "delimiter"() -> (w1034:string)
            n639 = property on="settings 4ch" class="Clust (strict)"(error in=w1031) -> (error out=w1029:errorcluster, "Value"=w1030:T21)  [unwired: 1 in, 1 out]
            n640 = call <instrlib>:"writeSettingsFile4ch.vi"("delimiter (,)"=w1034, "error in (no error)"=w1036, "old settings"=w1040, "new settings"=w1030, "path"=w1035) -> ("error out"=w1037:errorcluster)  [unwired: 5 in, 1 out]
            n641 = property on="settings_old" class="Clust (strict)"(error in=w1029, "Value"=w1030) -> ()  [unwired: 1 in, 2 out]
            n642 = call <vilib>:"Release Semaphore.vi"("error in (no error)"=w1037, "semaphore"=w1038) -> ()  [unwired: 4 in, 2 out]
          }
          frame "start acquisition" {
            w1093 = connectionState."acquiring data" ("connection state")
            n643 = local read "device type"() -> (w1081:T6)
            n644 = local read "dataTable"() -> (w1095:string[][])
            n645 = Empty Array?(array=w1095) -> (empty?=w1094:bool)
            n646 = local read "ref ctrls"() -> (w1092:T1)
            n647 = local write "connection state"(w1093) -> ()
            n648 = case shown="True" w1094 {
              tunnel: ["Acquisition started." "Acquisition started. Current time is 0s."] -> w1090
              tunnel: [w1096 w1099] -> w1089
              frame False {
                n649 = Get Date/Time In Seconds() -> (seconds since 1Jan1904=w1096:timestamp)
              }
              frame True {
                n650 = local read "timer-begin"() -> (w1099:timestamp)
              }
            }
            n651 = call <instrlib>:"controlVisibility4Ch.vi"("device type [AB1004]"=w1081, "ref controls"=w1092, "connection state"=w1093) -> ()  [unwired: 9 in]
            n652 = call <vilib>:"Acquire Semaphore.vi"("semaphore"=w1083) -> ("error out"=w1088:errorcluster, "semaphore out"=w1087:T13)  [unwired: 4 in, 1 out]
            n653 = property on="path-settings" class="Path"(error in=w1088) -> (error out=w1085:errorcluster, "Value"=w1084:path)  [unwired: 1 in, 1 out]
            n654 = local read "delimiter"() -> (w1082:string)
            n655 = call <instrlib>:"prependTimestamp.vi"("string in"=w1090) -> ("string out"=w1091:string)  [unwired: 14 in]
            n656 = call <instrlib>:"writeSettingsFile4ch.vi"("delimiter (,)"=w1082, "message (overrides settings)"=w1090, "timestamp (current)"=w1089, "error in (no error)"=w1085, "path"=w1084) -> ("error out"=w1086:errorcluster)  [unwired: 5 in, 1 out]
            n657 = local write "status"(w1091) -> ()
            n658 = call <vilib>:"Release Semaphore.vi"("error in (no error)"=w1086, "semaphore"=w1087) -> ()  [unwired: 4 in, 2 out]
          }
          frame "stop acquisition" {
            w1108 = "Acquisition stopped."
            n659 = local read "connection state"() -> (w1111:T8)
            n660 = case shown="\"acquiring data\", Default" w1111 {
              selector: w1111 -> [_ w1115 w1116]
              tunnel: [connectionState."connected" ("connection state") w1115 w1116] -> w1110
              tunnel: w1108 -> [w1112 _ _]
              frame "acquiring data", Default {
                n661 = call <instrlib>:"prependTimestamp.vi"("string in"=w1112) -> ("string out"=w1113:string)  [unwired: 14 in]
                n662 = local write "status"(w1113) -> ()
              }
              frame "connection error" {
              }
              frame "acquisition error" {
              }
            }
            n663 = call <vilib>:"Acquire Semaphore.vi"("semaphore"=w1102) -> ("error out"=w1107:errorcluster, "semaphore out"=w1106:T13)  [unwired: 4 in, 1 out]
            n664 = local read "delimiter"() -> (w1101:string)
            n665 = property on="path-settings" class="Path"(error in=w1107) -> (error out=w1104:errorcluster, "Value"=w1103:path)  [unwired: 1 in, 1 out]
            n666 = call <instrlib>:"writeSettingsFile4ch.vi"("delimiter (,)"=w1101, "message (overrides settings)"=w1108, "error in (no error)"=w1104, "path"=w1103) -> ("error out"=w1105:errorcluster)  [unwired: 6 in, 1 out]
            n667 = local write "connection state"(w1110) -> ()
            n668 = local read "ref ctrls"() -> (w1109:T1)
            n669 = call <vilib>:"Release Semaphore.vi"("error in (no error)"=w1105, "semaphore"=w1106) -> ()  [unwired: 4 in, 2 out]
            n670 = local read "device type"() -> (w1100:T6)
            n671 = call <instrlib>:"controlVisibility4Ch.vi"("device type [AB1004]"=w1100, "ref controls"=w1109, "connection state"=w1110) -> ()  [unwired: 9 in]
          }
          frame "unlock settings" {
            n672 = local read "device type"() -> (w1119:T6)
            n673 = property on="butUnlockSett" class="Bool"("Visible"=FALSE) -> (error out=w1117:errorcluster)  [unwired: 2 in, 1 out]
            n674 = case shown="1002, 1502, 1902, 2002, 2502" w1119 {
              tunnel: T17."Enabled" ("Disabled") -> [w1122 w1123]
              frame 1004, 1504, 1904, 2004, 2504, Default {
                n675 = property on="settings 4ch" class="Clust (strict)"("DisabledEnum"=w1122) -> ()  [unwired: 2 in, 2 out]
              }
              frame 1002, 1502, 1902, 2002, 2502 {
                n676 = property on="settings 2ch" class="Clust (strict)"("DisabledEnum"=w1123) -> ()  [unwired: 2 in, 2 out]
              }
            }
            n677 = property on="butLoadDefSett" class="Bool"(error in=w1117, "Visible"=TRUE) -> ()  [unwired: 1 in, 2 out]
          }
          frame Default {
          }
        }
      }
      frame Error {
        # "Return true in any case that should stop the loop."
      }
    }
  }
  n678 = while {
    tunnel: w15 -> [w1133]
    tunnel: w17 -> [w1129]
    tunnel: w16 -> [w1128]
    stop <- w1132 stop-if-true
    # "read sample loop"
    n679 = Wait on Notification(notifier=w1133, ignore previous (F)=TRUE) -> (notification=w1131:timestamp, error out=w1125:errorcluster)  [unwired: 2 in, 2 out]
    n680 = local read "error"() -> (w1127:errorcluster)
    n681 = Merge Errors(w1125, w1127) -> (w1126:errorcluster)
    n682 = case shown="No Error" w1126 {
      tunnel: [FALSE w1158] -> w1132
      tunnel: w1131 -> [w1150 _]
      tunnel: w1129 -> [w1152 _]
      tunnel: w1128 -> [w1151 _]
      tunnel: w1125 -> [_ w1159]
      frame No Error {
        n683 = local read "abacus VISA"() -> (w1145:refnum<visa-resource-name>)
        n684 = local read "device type"() -> (w1134:T6)
        n685 = call <vilib>:"Acquire Semaphore.vi"("semaphore"=w1151) -> ("error out"=w1147:errorcluster, "semaphore out"=w1149:T13)  [unwired: 4 in, 1 out]
        n686 = call <instrlib>:"Read Measurement.vi"("device type"=w1134, "error in (no error)"=w1147, "read timeout (500 ms)"=u32 250 ("read timeout (10000 ms)"), "VISA Refnum in"=w1145) -> ("error out"=w1146:errorcluster, "values"=w1136:u32[], "labels"=w1137:string[], "read time"=w1143:timestamp)  [unwired: 2 in, 2 out]
        "timer-lastRead" <- w1143
        n687 = property on="error" class="Clust (strict)"("Val(Sgnl)"=w1146) -> (error out=w1148:errorcluster)  [unwired: 2 in, 1 out]
        n688 = call <instrlib>:"Bundle by Name Data 4ch.vi"("names"=w1137, "values"=w1136) -> ("output cluster 4ch"=w1135:T11)  [unwired: 13 in]
        n689 = call <vilib>:"Release Semaphore.vi"("error in (no error)"=w1148, "semaphore"=w1149) -> ()  [unwired: 4 in, 2 out]
        n690 = Unbundle By Name(w1135) -> ("counters_ID"=w1138:u32)
        n691 = Unbundle By Name(w1135) -> ("time_left"=w1140:u32)
        n692 = Divide(x=w1140, y=1000.0) -> (x/y=w1139:dbl)
        n693 = case shown="1.." w1138 {
          tunnel: w1152 -> [w1157 _]
          tunnel: w1135 -> [w1156 _]
          tunnel: w1143 -> [w1155 _]
          frame 1.. {
            n694 = Bundle("read time"=w1155, "output cluster 4ch"=w1156) -> (w1154:T24)  [unwired: 1 in]
            n695 = Enqueue Element "adds data in queue"(queue=w1157, element=w1154) -> ()  [unwired: 2 in, 3 out]
          }
          frame 0, Default {
            # "ID=0 means\ninvalid data"
          }
        }
        n696 = Add(x=w1143, y=w1139) -> (x+y=→"timer-nextRead":timestamp)
        "timer-readRequest" <- w1150
      }
      frame Error {
        n697 = Unbundle By Name(w1159) -> ("status"=w1158:bool)
      }
    }
  }
  n698 = while {
    tunnel: w14 -> [w1166]
    tunnel: w12 -> [w1164]
    shift-right: [w1163] -> _
    shift-left: w2 -> [w1162]
    shift-right: [w1160] -> _
    shift-left: w1 -> [w1161]
    stop <- w1168 stop-if-true
    w1167 = u32 250  # refresh rate
    # "update dataGUI and datafile loop"
    n699 = Dequeue Element(queue=w1166) -> (queue out=w1165:refnum<queue>, element=w1170:T15, error out=w1169:errorcluster)  [unwired: 2 in, 1 out]
    n700 = Wait (ms)(milliseconds to wait=w1167) -> ()  [unwired: 1 out]
    n701 = case shown="No Error" w1169 {
      selector: w1169 -> [w1210 _]
      tunnel: w1170 -> [w1209 _]
      tunnel: [FALSE TRUE] -> w1168
      tunnel: w1165 -> [w1211 _]
      tunnel: w1164 -> [w1203 _]
      tunnel: [w1180 w1214] -> w1163
      tunnel: w1162 -> [w1189 w1214]
      tunnel: w1161 -> [w1175 w1213]
      tunnel: [w1174 w1213] -> w1160
      frame No Error {
        w1181 = 100  # data in graphs
        n702 = Flush Queue(queue=w1211, error in (no error)=w1210) -> (remaining elements=w1208:T12)  [unwired: 2 out]
        n703 = local read "timer-begin"() -> (w1192:timestamp)
        n704 = local read "device type"() -> (w1171:T6)
        n705 = Build Array (concatenate)(w1209, w1208) -> (w1205:T12)
        n706 = Reverse 1D Array "most\nrecent first"(array=w1205) -> (reversed array=w1190:T12)
        n707 = call <instrlib>:"timestampAndDataToTable 4ch.vi"("device type [AB1004]"=w1171, "data in"=w1190, "session start timestamp"=w1192) -> ("table data"=w1173:string[][], "table headers"=w1191:string[])  [unwired: 6 in, 1 out]
        n708 = local read "delimiter"() -> (w1195:string)
        n709 = Index Array "get most\nrecent value"(array=w1190, index=0) -> (element=w1206:T15)
        n710 = property on="dataTable" class="Tbl (strict)"("Column Headers[]"=w1191) -> ()  [unwired: 2 in, 2 out]
        n711 = Build Array (concatenate) "prepend new data"(w1190, w1189) -> (w1182:T12)
        n712 = Build Array (concatenate) "prepend new data"(w1173, w1175) -> (w1174:string[][])
        "dataTable" <- w1174
        n713 = call <vilib>:"reverse 2D array.vi"("Previously Selected List"=w1173) -> ("All Items List"=w1172:string[][])
        n714 = call <vilib>:"Acquire Semaphore.vi"("semaphore"=w1203) -> ("error out"=w1201:errorcluster, "semaphore out"=w1204:T13)  [unwired: 4 in, 1 out]
        n715 = Unbundle(w1206) -> ("counters 4ch"=w1194:T11)  [unwired: 1 out]
        "counters 4ch" <- w1194
        n716 = property on="path-file" class="Path"(error in=w1201) -> (error out=w1200:errorcluster, "Value"=w1199:path)  [unwired: 1 in, 1 out]
        n717 = call <instrlib>:"Counters4ch To Counters2ch.vi"("counters4ch"=w1194) -> ("counters2ch"=→"counters 2ch":T10)
        n718 = Array Subset "extract\nrecent data"(array=w1182, length=w1181) -> (w1180:T12)  [unwired: 1 in]
        n719 = call-poly <vilib>:"Write Delimited Spreadsheet.vi"("file path (dialog if empty)"=w1199, "2D data"=w1172, "append to file? (F)"=TRUE, "error in (no error)"=w1200, "delimiter (\\t)"=w1195) -> ("new file path (Not A Path if cancelled)"=w1198:path, "error out"=w1197:errorcluster)  [unwired: 9 in]
        n720 = property on="path-file" class="Path"(error in=w1197, "Value"=w1198) -> (error out=w1196:errorcluster)  [unwired: 1 in, 1 out]
        n721 = call <instrlib>:"data to graphs.vi"("data in"=w1180) -> ("graph coincidences"=→"graph coinc":cluster{timestamp[], u32[]}[], "graph singles"=w1187:cluster{timestamp[], u32[]}[])  [unwired: 9 in]
        n722 = call <vilib>:"Release Semaphore.vi"("error in (no error)"=w1196, "semaphore"=w1204) -> ()  [unwired: 4 in, 2 out]
        n723 = Index Array(array=w1187, index #1=0 ("index"), index #2=1 ("index"), index #3=2 ("index"), index #4=3 ("index")) -> (element #1=→"graph-A-S" →"graph-A":cluster{timestamp[], u32[]}, element #2=→"graph-B-S" →"graph-B":cluster{timestamp[], u32[]}, element #3=→"graph-C-S" →"graph-C":cluster{timestamp[], u32[]}, element #4=→"graph-D-S" →"graph-D":cluster{timestamp[], u32[]})
      }
      frame Error {
      }
    }
  }
  n724 = Unbundle(w6) -> ("semaphore files"=w28:T13, "semaphore port"=w27:T13, "notifier read request"=w22:refnum<notifier>, "queue data"=w25:refnum<queue>, "queue instructions"=w26:refnum<queue>)
  n725 = Release Queue(queue=w26, error in (no error)=w21) -> (error out=w43:errorcluster)  [unwired: 1 in, 2 out]
  n726 = Release Queue(queue=w25, error in (no error)=w43) -> (error out=w24:errorcluster)  [unwired: 1 in, 2 out]
  n727 = Release Notifier(notifier=w22, error in (no error)=w24) -> (error out=w23:errorcluster)  [unwired: 1 in, 2 out]
  n728 = call <vilib>:"Release Semaphore Reference.vi"("error in (no error)"=w23, "semaphore"=w27) -> ("error out"=w33:errorcluster)  [unwired: 8 in, 1 out]
  n729 = call <vilib>:"Release Semaphore Reference.vi"("error in (no error)"=w33, "semaphore"=w28) -> ("error out"=w10:errorcluster)  [unwired: 8 in, 1 out]
  n730 = disable-structure shown="RUN_TIME_ENGINE==True" {
    disable-tunnel: w10 -> [_ _]
    frame condition #0 (active) {
    }
    frame condition #1 {
      n731 = Quit LabVIEW() -> ()  [unwired: 1 in]
    }
  }
